vi "Create_Trajectory_Using_TrajectoryLibraryXXX.vi"() -> ()   [LabVIEW 2019]
doc: "This utility creates trajectories based on the robot configuration, constraints and defined waypoints."
uses:
  <vilib>/Rock Robotics/WPI/ThirdParty/JAS_Junk/TrajLib/TypeDef/DISPLAY_WEIGHTED_WAYPOINT.ctl
  <vilib>/Rock Robotics/WPI/ThirdParty/JAS_Junk/TrajLib/TypeDef/TRAJ_STATE.ctl
  <vilib>/Rock Robotics/WPI/ThirdParty/JAS_Junk/TrajLib/TypeDef/POSE2D.ctl
  <vilib>/Rock Robotics/WPI/ThirdParty/JAS_Junk/TrajLib/TypeDef/TRANSLATION2D.ctl
  <vilib>/Rock Robotics/WPI/ThirdParty/JAS_Junk/TrajLib/TypeDef/ROTATION2D.ctl
  <vilib>/Rock Robotics/WPI/ThirdParty/JAS_Junk/TrajLib/TypeDef/SIMPLE_MOTOR_FF.ctl
  CreateTrajectoryENUM/TrajCreateUnitsENUM.ctl
  <vilib>/Rock Robotics/WPI/ThirdParty/JAS_Junk/TrajLib/TypeDef/TRAJECTORY.ctl
  <vilib>/Rock Robotics/WPI/ThirdParty/JAS_Junk/TrajLib/TypeDef/TRAJ_CONFIG.ctl
  <vilib>/vision/Image Controls.llb/IMAQ Image.ctl
  <vilib>/Rock Robotics/WPI/ThirdParty/JAS_Junk/TrajLib/TypeDef/TRAJ_CONSTRAINT_RECT_REGION.ctl
  <vilib>/Rock Robotics/WPI/ThirdParty/JAS_Junk/TrajLib/Enum/TRAJ_CONSTRAINT_TYPES_ENUM.ctl
  <vilib>/Utility/miscctls.llb/LVCursorListTypeDef.ctl
  CreateTrajectoryTypeDef/TrajCreateConfig__V_Internal.ctl
  <vilib>/Rock Robotics/WPI/ThirdParty/JAS_Junk/TrajLib/Conv_Inches_Meters.vi
  <vilib>/Rock Robotics/WPI/ThirdParty/JAS_Junk/TrajLib/Conv_Feet_Meters.vi
  <vilib>/Rock Robotics/WPI/ThirdParty/JAS_Junk/TrajLib/Conv_Meters_Inches.vi
  <vilib>/Rock Robotics/WPI/ThirdParty/JAS_Junk/TrajLib/Conv_Meters_Feet.vi
  <vilib>/Rock Robotics/SystemInterfaces/NetworkCommunication/NetComm_UsageReport_report.vi
  <vilib>/Rock Robotics/WPI/ThirdParty/JAS_Junk/TrajLib/CentripetalAccelConstraint_New.vi
  <vilib>/Rock Robotics/WPI/ThirdParty/JAS_Junk/TrajLib/DiffDriveVoltageConstraint_New.vi
  <vilib>/Rock Robotics/WPI/ThirdParty/JAS_Junk/TrajLib/SwerveDriveKinematicsConstraint_New.vi
  <vilib>/Rock Robotics/WPI/ThirdParty/JAS_Junk/TrajLib/MecaDriveKinematicsConstraint_New.vi
  <vilib>/Rock Robotics/WPI/ThirdParty/JAS_Junk/TrajLib/VI/TrajConstraint_GetType.vi
  <vilib>/Utility/xml.llb/Read From XML File(string).vi
  <vilib>/Utility/Data Type/Get Type Information.vi
  <vilib>/Utility/xml.llb/Write to XML File(string).vi
  <vilib>/Rock Robotics/WPI/ThirdParty/JAS_Junk/TrajLib/Globals/Util_LibraryGlobals.vi
  <vilib>/Rock Robotics/WPI/ThirdParty/JAS_Junk/TrajLib/Trajectory_Library.lvlib
panel:
  out "value":T1={"BottomLeftPoint"={"X"=0.0, "Y"=0.0}, "TopRightPoint"={"X"=0.0, "Y"=0.0}, "Constraint"=variant, "Constraint Type"=enum."DIFF DRIVE KINEMATICS"} {"TopRightPoint"."Y" format="%14.3f"; "TopRightPoint"."X" format="%14.3f"; "BottomLeftPoint"."Y" format="%14.3f"; "BottomLeftPoint"."X" format="%14.3f"}
  out "error out 2":errorcluster
  out "LabVIEW Data":variant
  out "error out":errorcluster
  out "xml string":string
  in  "Terminate":bool
  out "FIeld Image":T4
  out "FIeldSelectorHasItems":bool
  out "IsCubic":bool
  out "outTRAJECTORY_CONFIG":T5 {"End Velocity" format="%20.4f"; "StartVelocity" format="%20.4f"; "Max Acceleration" format="%20.4f"; "MaxVelocity" format="%20.4f"}
  out "WayPoints_M":T6[](array[typedef]) {"WEIGHT" format="%13.3f"; "ANGLE" format="%13.3f"; "Y" format="%13.3f"; "X" format="%13.3f"}
  out "TRAJECTORY":T7 {"States"."POSE"."ROTATION"."SIN" format="%13.4f"; "States"."POSE"."ROTATION"."COS" format="%13.4f"; "States"."POSE"."ROTATION"."VALUE" format="%13.4f"; "States"."POSE"."TRANSLATION"."Y" format="%14.3f"; "States"."POSE"."TRANSLATION"."X" format="%14.3f"; "TotalTImeSecs" format="%20.3f"}
  in  "End Program":bool
  in  "Tab Control":T11(tab)
  out "Config File Read\nWithout Error":bool
  out "Config File  Read Error":errorcluster
  out "Read Config File Comment":string
  in  "Read Config File Name":path
  in  "ReadConfigFile":bool
  in  "Field Selector":string(combo)
  in  "Units Selector":T12
  in  "MaxVelocity":dbl=50.0 format="%17.1f"
  in  "MaxAcceleration":dbl=40.0 format="%17.1f"
  out "MaxVelocity M/S":dbl=2.0 format="%17.4f"
  out "MaxAcceleration M/S^2":dbl=1.3 format="%17.4f"
  in  "Right Rear":T2={"X"=-0.5, "Y"=0.5} {"Y" format="%14.3f"; "X" format="%14.3f"}
  in  "Left Rear":T2={"X"=-0.5, "Y"=-0.5} {"Y" format="%14.3f"; "X" format="%14.3f"}
  in  "Right Front":T2={"X"=0.5, "Y"=0.5} {"Y" format="%14.3f"; "X" format="%14.3f"}
  in  "Left Front":T2={"X"=0.5, "Y"=-0.5} {"Y" format="%14.3f"; "X" format="%14.3f"}
  in  "Use Centripetal\nAcceleration\nConstaint":bool=TRUE
  out "Max Cent Accel M/S^2":dbl=1.0 format="%20.4f"
  in  "Max Cent Accel":dbl=20.0 format="%20.1f"
  in  "Use Diff Drive\nKinematic\nConstraint":bool=TRUE
  out "Track Width M":dbl=0.66 format="%20.4f"
  in  "Track Width":dbl=20.866 format="%20.1f"
  in  "Max Voltage":dbl=12.0 format="%20.4f"
  in  "SIMPLE_MOTOR_FF":T13={"Ks"=0.9, "Kv"=0.22199, "Ka"=0.04876, "KnInv"=1.0} {"KnInv" format="%13.4f"; "Ka" format="%13.4f"; "Kv" format="%13.4f"; "Ks" format="%13.4f"}
  in  "Use Diff Drive\nVoltage\nConstraint":bool
  in  "Wheels":T2[](array[typedef])=[{"X"=0.5, "Y"=-0.5}, {"X"=0.5, "Y"=0.5}, {"X"=-0.5, "Y"=0.5}, {"X"=-0.5, "Y"=-0.5}] {"Y" format="%14.3f"; "X" format="%14.3f"}
  in  "Use Swerve Drive\nKinematics\nConstraint":bool
  in  "Use Mecanum \nDrive Kinematics\nConstraint":bool
  out "Left Front M":T2 {"Y" format="%14.3f"; "X" format="%14.3f"}
  out "Right Front M":T2 {"Y" format="%14.3f"; "X" format="%14.3f"}
  out "Left Rear M":T2 {"Y" format="%14.3f"; "X" format="%14.3f"}
  out "Right Rear M":T2 {"Y" format="%14.3f"; "X" format="%14.3f"}
  out "SIMPLE_MOTOR_FF M":T13={"Ks"=0.0, "Kv"=0.0, "Ka"=0.0, "KnInv"=1.0} {"KnInv" format="%13.4f"; "Ka" format="%13.4f"; "Kv" format="%13.4f"; "Ks" format="%13.4f"}
  out "Wheels M":T2[](array[typedef]) {"Y" format="%14.3f"; "X" format="%14.3f"}
  in  "Use Rectangular Region\nDiff Drive Kinematics\nConstraint":bool
  in  "Rect Reg Top Right":T2 {"Y" format="%14.3f"; "X" format="%14.3f"}
  in  "REct Reg Bot Left":T2 {"Y" format="%14.3f"; "X" format="%14.3f"}
  in  "Max Speed (Units/Sec)":dbl=40.0 format="%20.4f"
  in  "Max Accel (Units/Sec^2)":dbl=100.0 format="%20.4f"
  out "Rect Reg Top Right M":T2 {"Y" format="%14.3f"; "X" format="%14.3f"}
  out "Rect Reg Bot Left M":T2 {"Y" format="%14.3f"; "X" format="%14.3f"}
  out "Max Sped M/Sec":dbl
  out "Max Accel M/Sec^2":dbl
  in  "Remove Current\nWaypoint":bool
  in  "Add New\nWaypoint":bool
  in  "WayPoints":T6[](array[typedef])=[{"X"=15.0, "Y"=105.0, "ANGLE"=-45.0, "WEIGHT"=12.0}, {"X"=105.0, "Y"=65.0, "ANGLE"=0.0, "WEIGHT"=12.0}, {"X"=210.0, "Y"=106.0, "ANGLE"=45.0, "WEIGHT"=12.0}, {"X"=350.0, "Y"=105.0, "ANGLE"=-45.0, "WEIGHT"=12.0}] {"WEIGHT" format="%13.3f"; "ANGLE" format="%13.3f"; "Y" format="%13.3f"; "X" format="%13.3f"}
  in  "Spline Type":enum32{"Radio Selection 1", "Radio Selection 2"}(radio)
  in  "Reverse":bool
  in  "UseWeights":bool
  in  "Calculate\nTrajectory":bool
  out "Trajectory\nCompleted\nError Free":bool
  out "Trajectory calculation error":errorcluster
  out "Position":cluster{dbl[], dbl[]}[](graph)
  out "Field Display":T4(plugin-control)
  out "Index":i32
  out "Trajectory Data":cluster{dbl[], dbl[]}[](graph)
  out "differential \ndrive \nmax speed":dbl format="%15.1f"
  out "Traj States\nSize":i32
  out "Trajectory States":T8[](array[typedef]) {"POSE"."ROTATION"."SIN" format="%13.4f"; "POSE"."ROTATION"."COS" format="%13.4f"; "POSE"."ROTATION"."VALUE" format="%13.4f"; "POSE"."TRANSLATION"."Y" format="%14.3f"; "POSE"."TRANSLATION"."X" format="%14.3f"}
  in  "Trajectory JSON File Name":path
  out "JSON File Saved\nWithout Error":bool
  out "Write CSV File Error":errorcluster
  in  "PathWeaver Length Units":T14(radio)
  in  "WriteJSONFile":bool
  out "CSV File Saved\nWithout Error":bool
  in  "Trajectory Type":enum32{"Radio Selection 1", "Radio Selection 2"}(radio)
  out "Write Trajectory\nFile Error":errorcluster
  in  "Trajectory File Comment":string
  in  "Trajectory CSV File Name":path
  in  "WriteTrajFile":bool
  out "Config File Saved\nWithout Error":bool
  out "Write Config FIle Error":errorcluster
  in  "Write Config File Comment":string
  in  "Write Config File Name":path
  in  "WriteConfigFile":bool
  # "Create Trajectory  (Use LabVIEW trajectory library)"
  # "Instructions:  \n----------------\n\nThis utility will create a trajectory, show the data on the various tabs, and optionally write a \"field absolute\" or \"robot relative\" trajectory to a file. \nTo use this utility:\n\n    1) Read all of these instructions!\n    2) Define the robot's physical data on the \"Robot Data\" tab.  \n    3) Define the robot's movement constraints on the \"Constraints\" page.  \n    4) Define the trajectory on the \"Define/Create Trajectory\" tab.  These are the beginning and ending positions/headings, and internal positions/headings.  \n         Cubic splines only use the first and last \"angle\".  The other internal \"angles\" are calculated.  Quintic splines use all the defined angles.\n    5) Press the \"Calculate Trajectory\".  If a good trajectory was calculated it will be displayed.  If no errors are generated the Trajectory Complete\n         light will be on.  Errors will be displayed in the error indicator.  The path can be recalculated many times before performing any other action.\n\nAfter a Trajectory has been calculated, the \"trajectory can be written to a file.  The absolute path is converted to a robot relative trajectory.  To do this:\n    1) Enter a comment to be included in the file.  Anything can be entered.\n    2) Select the file name.\n    3) Press \"Create Trajectory File\"  If an error occurs it will be displayed in the File Creation Error indicator.\n\nTo:\n  --  Move a WayPoint  -- Left click the waypoint and drag it using the mouse.\n  --  Rotate a WayPoint  -- Left click the waypoint to select, then use the mouse wheel to increase or decrease the heading\n  --  Change WayPoint weight  -- Left click the waypoint to select, then use CTRL key and mouse wheel to increase or decrease the weight.\n\nNotes:\n--------\n- All the robot parameters, path, and field dimensions are in UNITS, and DEGREES.  Select UNITS from the \"Robot Data\" page.  The resulting  \n  trajectory is converted to METERS, and RADIANS to match the rest of this library!\n- The trajectory library is the same as the WPILIB spline and trajectory library for Java and C++.\n- 2019 playing field size - width: 26 ft 11.25 In = 323.25 in , length: 52 ft 5.25 in = 629.25 in  (I didn't verify this for the 2020 version.)\n\nAcknowlegements\n------------------------\n- Nathanael Cornell from FRC team 5205 added the initial code to visually move and rotate waypoints."
  # "Read Trajectory Waypoints and Configuration from File"
  # "ROBOT DATA"
  # "UNITS/SEC"
  # "Meters/SEC"
  # "UNITS/SEC^2"
  # "Meters/SEC^2"
  # "Simulated robot max speed is: 68.266 Inches/Second"
  # "UTILITY CONFIGURATION"
  # "Diff Kinematics Constraint"
  # "Centripetal Accel Constraint"
  # "Diff Voltage Constraint"
  # "UNITS"
  # "UNITS/SEC^2"
  # "VOLTS"
  # "METERS"
  # "METERS/SEC^2"
  # "Distance is:\nUNITS"
  # "Simulated robot wheelbase is 20.87 in"
  # "Ks = Volts\nKv = VoltSec/Meter\nKa = Volt(Sec^2)/Meter"
  # "Swerve Kinematics Constraint"
  # "Mechanum Kinematics Constraint"
  # "Values\nare \nUNITS"
  # "Values\nare \nUNITS"
  # "Rectangular Region Constraint  - Diff Drive Constraint"
  # "Values\nare \nUNITS"
  # "TRAJECTORY DEFINITION"
  # "To delete array elements or the entire array, right click on the array or element, select Data Operations, then select the action to be performed."
  # "UNITS, UNITS, DEGREES, SCALAR"
  # "INCHES/SEC"
  # "Write Trajectory to File   -   CSV, and / or JSON"
  # "Write Trajectory Waypoints and Configuration to File"
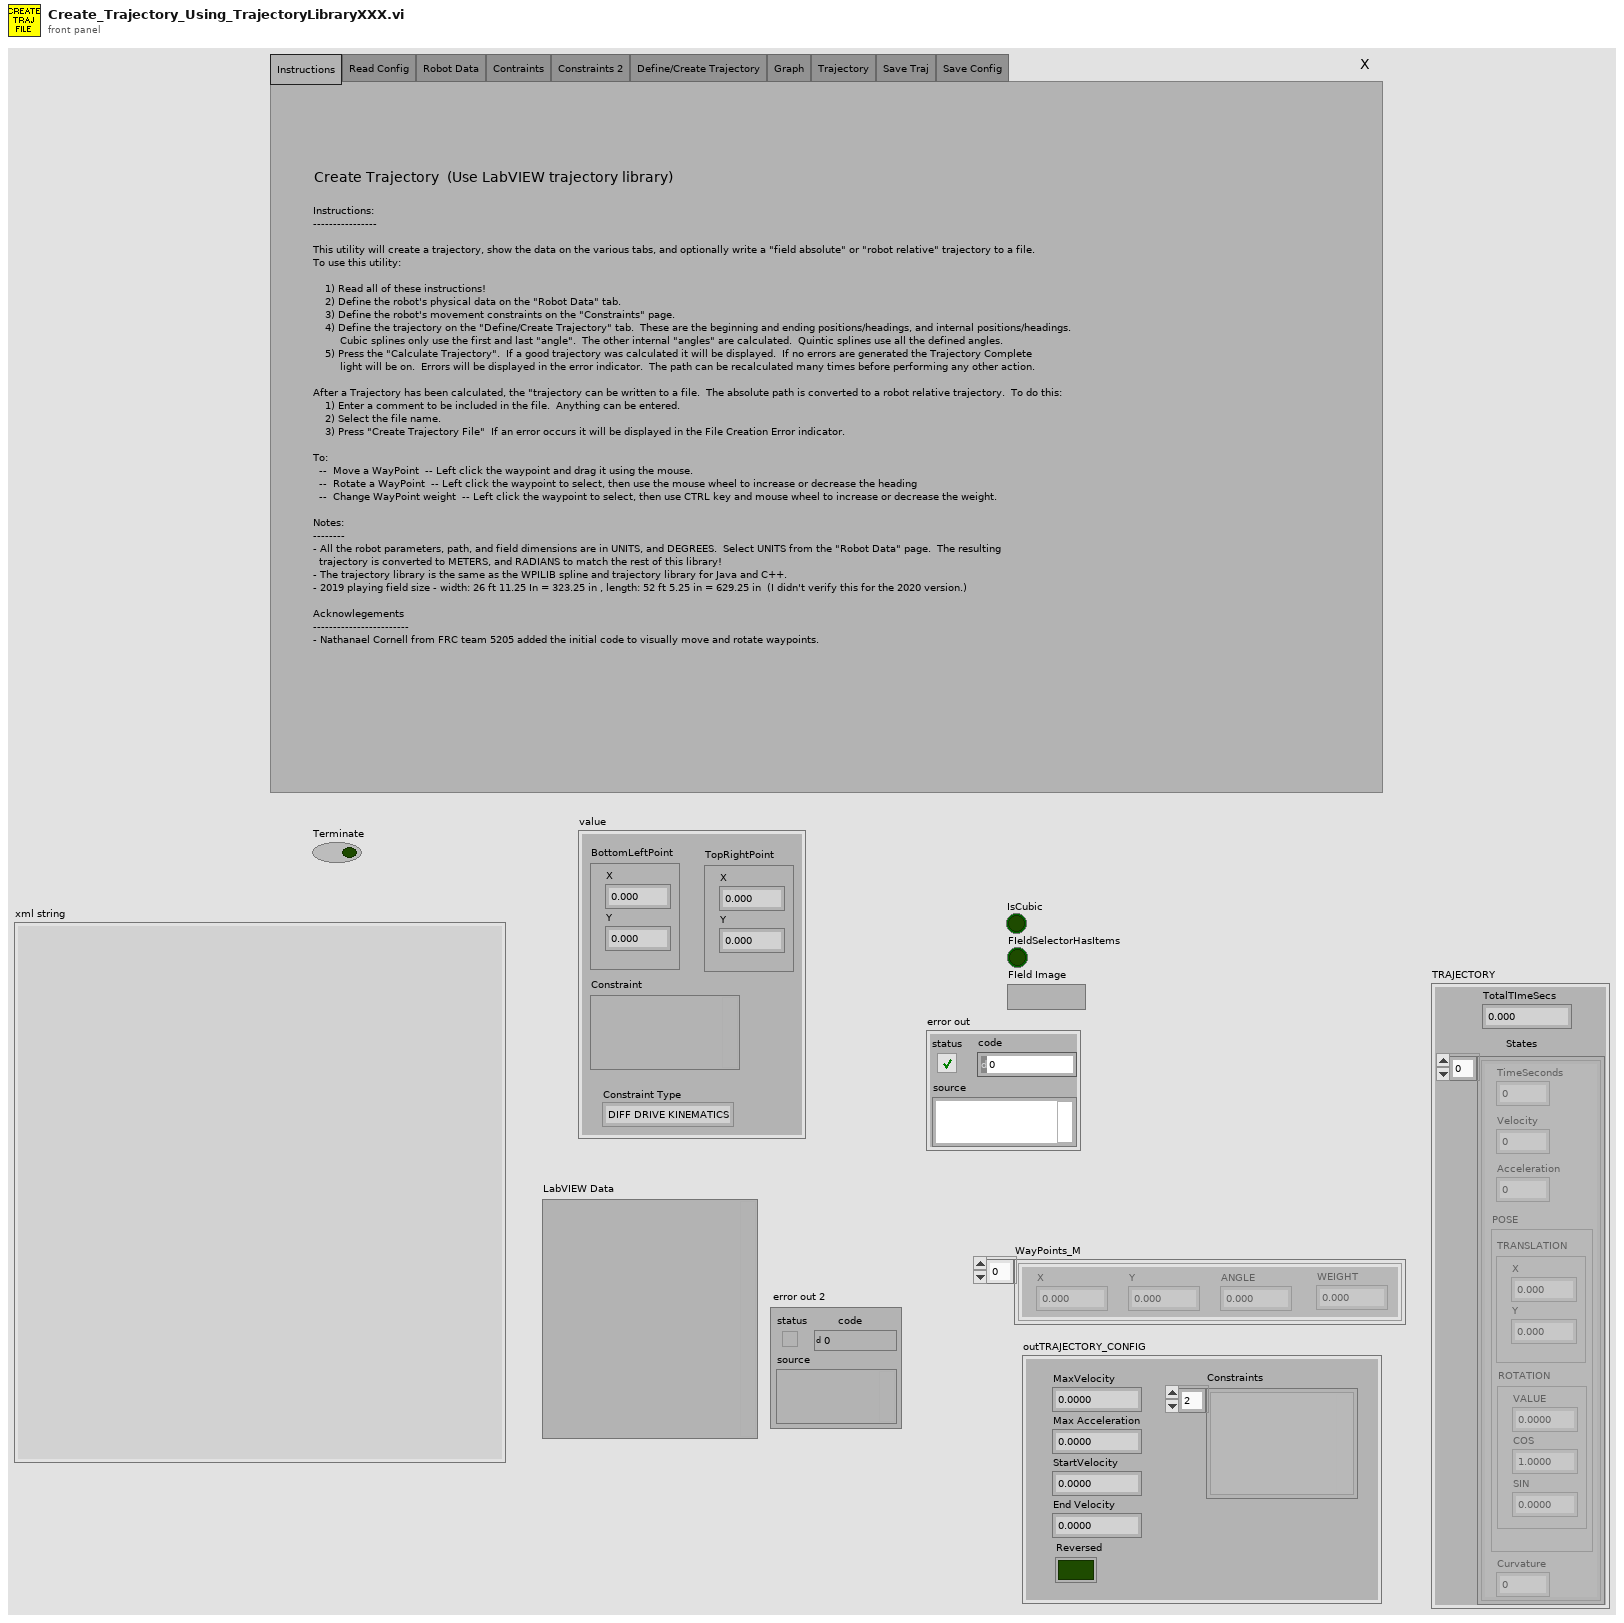
[diagram p1: front panel]
types:
  T1 = typedef "Trajectory_Library.lvlib/TRAJ_CONSTRAINT_RECT_REGION.ctl" = cluster{"BottomLeftPoint":T2, "TopRightPoint":T2, "Constraint":variant, "Constraint Type":T3}
  T2 = typedef "Trajectory_Library.lvlib/TRANSLATION2D.ctl" = cluster{"X":dbl, "Y":dbl}
  T3 = typedef "Trajectory_Library.lvlib/TRAJ_CONSTRAINT_TYPES_ENUM.ctl" = enum16{"UNDEFINED", "DIFF DRIVE KINEMATICS", "DIFF DRIVE VOLTAGE", "CENTRIPITAL ACCEL", "MECA DRIVE KINEMATICS", "SWERVE DRIVE KINEMATICS", "MAXIMUM VELOCITY", "ELLIPTICAL REGION", "RECTANGULAR REGION"}
  T4 = typedef "IMAQ Image.ctl" = refnum<image>
  T5 = typedef "Trajectory_Library.lvlib/TRAJ_CONFIG.ctl" = cluster{"MaxVelocity":dbl, "Max Acceleration":dbl, "StartVelocity":dbl, "End Velocity":dbl, "Reversed":bool, "Constraints":variant[]}
  T6 = typedef "Trajectory_Library.lvlib/DISPLAY_WEIGHTED_WAYPOINT.ctl" = cluster{"X":dbl, "Y":dbl, "ANGLE":dbl, "WEIGHT":dbl}
  T7 = typedef "Trajectory_Library.lvlib/TRAJECTORY.ctl" = cluster{"TotalTImeSecs":dbl, "States":T8[]}
  T8 = typedef "Trajectory_Library.lvlib/TRAJ_STATE.ctl" = cluster{"TimeSeconds":dbl, "Velocity":dbl, "Acceleration":dbl, "POSE":T9, "Curvature":dbl}
  T9 = typedef "Trajectory_Library.lvlib/POSE2D.ctl" = cluster{"TRANSLATION":T2, "ROTATION":T10}
  T10 = typedef "Trajectory_Library.lvlib/ROTATION2D.ctl" = cluster{"VALUE":dbl, "COS":dbl, "SIN":dbl}
  T11 = enum32{"Instructions", "Read Config", "Robot Data", "Contraints", "Constraints 2", "Define/Create Trajectory", "Graph", "Trajectory", "Save Traj", "Save Config"}
  T12 = typedef "TrajCreateUnitsENUM.ctl" = enum16{"Inches", "Feet", "Centimeters", "Meters"}
  T13 = typedef "Trajectory_Library.lvlib/SIMPLE_MOTOR_FF.ctl" = cluster{"Ks":dbl, "Kv":dbl, "Ka":dbl, "KnInv":dbl}
  T14 = enum32{"Radio Selection 1", "Radio Selection 2", "Radio Selection 3", "Radio Selection 4", "Radio Selection 5"}
  T15 = typedef "Image Type" = u32
  T16 = typedef "TrajectoryUtils_Field_Info.ctl" = cluster{"FIeld_File_Name":string, "Top_Left_X":i32, "Top_Left_Y":i32, "Bottom_Right_X":i32, "Bottom_Right_Y":i32, "Field_Size_X":dbl, "Field_Size_Y":dbl, "FIeld_Size_Units":string}
  T17 = typedef "LVCursorListTypeDef.ctl" = cluster{"Name":string, "Color":u32, "Style":u8, "Point Style":u8, "Name Visible":bool, "Allow Drag":bool, "Cursor Mode":u32, "Plot":i32, "Index":i32, "Position":cluster{"X":dbl, "Y":dbl}, "X Scale":u32, "Y Scale":u32, "Watch Plots":i32[], "Watch All Plots":bool, "Plot Area":i32, "Label Offset":cluster{"X":dbl, "Y":dbl}}[]
  T18 = enum8{"Enabled", "Disabled", "Disabled and Grayed Out"}
  T19 = cluster{"Name":string, "Color":u32, "Style":u8, "Point Style":u8, "Name Visible":bool, "Allow Drag":bool, "Cursor Mode":u32, "Plot":i32, "Index":i32, "Position":cluster{"X":dbl, "Y":dbl}, "X Scale":u32, "Y Scale":u32, "Watch Plots":i32[], "Watch All Plots":bool, "Plot Area":i32, "Label Offset":cluster{"X":dbl, "Y":dbl}}
  T20 = typedef "TrajCreateConfig__V_Internal.ctl" = cluster{"Write Config File Name":path, "Write Config File Comment":string, "WayPoints":T6[], "TRAJECTORY_CONFIG":T5, "IsCubic":bool, "Units Selector":T12, "UseWeights":bool, "FieldName":string}
  T21 = typedef "Trajectory_Library.lvlib/TRAJ_CONSTRAINT_DIIF_DRIVE_KINEMATICS.ctl" = cluster{"Max Speed (M/S)":dbl, "DIFF_DRIVE_KINEMATICS":T22, "Max Accel (M/S2)":dbl}
  T22 = typedef "Trajectory_Library.lvlib/DIFF_DRIVE_KINEMATICS.ctl" = cluster{"TrackWidth_Meters":dbl}
  T23 = typedef "Trajectory_Library.lvlib/TRAJ_CONSTRAINT_CENTRIPETAL_ACCEL.ctl" = cluster{"Max Cent Accel":dbl}
  T24 = typedef "Trajectory_Library.lvlib/TRAJ_CONSTRAINT_DIIF_DRIVE_VOLTAGE.ctl" = cluster{"Max Voltage":dbl, "DIFF_DRIVE_KINEMATICS":T22, "SIMPLE_MOTOR_FF":T13}
  T25 = typedef "Trajectory_Library.lvlib/TRAJ_CONSTRAINT_MECA_DRIVE_KINEMATICS.ctl" = cluster{"Max Speed (M/S)":dbl, "MECA_DRIVE_KINEMATICS":T26}
  T26 = typedef "Trajectory_Library.lvlib/MECA_DRIVE_KINEMATICS.ctl" = cluster{"FrontLeft":T2, "FrontRight":T2, "RearLeft":T2, "RearRight":T2, "InverseKinematics":T27, "ForwardKinematics":T27, "PrevCoR":T2}
  T27 = typedef "NI_Matrix.lvlib/RealMatrix.ctl" = dbl[][]
  T28 = typedef "Trajectory_Library.lvlib/TRAJ_CONSTRAINT_SWERVE_DRIVE_KINEMATICS.ctl" = cluster{"Max Speed (M/S)":dbl, "SwerveKinematics":T29}
  T29 = typedef "Trajectory_Library.lvlib/SWERVE_DRIVE_KINEMATICS.ctl" = cluster{"NumModules":i32, "InverseKinematics":T27, "ForwardKinematics":T27, "Modules":T2[], "PrevCoR":T2, "SavedModuleStates":T30[]}
  T30 = typedef "Trajectory_Library.lvlib/SWERVE_DRIVE_MODULE_STATE.ctl" = cluster{"Speed":dbl, "Angle":T10}
  T31 = typedef "TrajCreateConfig_V4.ctl" = cluster{"Write Config File Name":path, "Write Config File Comment":string, "WayPoints":T6[], "TRAJECTORY_CONFIG_V4":T32, "IsCubic":bool, "Units Selector":T12, "UseWeights":bool, "FieldName":string}
  T32 = typedef "TrajCreateTrajConfig_V4.ctl" = cluster{"MaxVelocity":dbl, "Max Acceleration":dbl, "StartVelocity":dbl, "End Velocity":dbl, "Reversed":bool, "DiffDrKineConstntDefined":bool, "CentAcellConstntDefined":bool, "DiffDrVoltConstntDefined":bool, "DIFF_DRIVE_KINE_CONSTRAINT":T21, "CENTRIPETAL_ACCEL_CONSTRAINT":T23, "SwerveDrKineConstntDefined":bool, "SWERVE_DRIVE_KINE_CONSTRAINT":T28, "DIFF_DRIVE_VOLTAGE_CONSTRAINT":T24, "MECANUM_DRIVE_KINE_CONSTRAINT":T25, "MecanumDrKineConstntDefined":bool}
  T33 = cluster{"Shift":bool, "Ctrl":bool, "Alt":bool, "Cmd":bool, "Opt":bool}
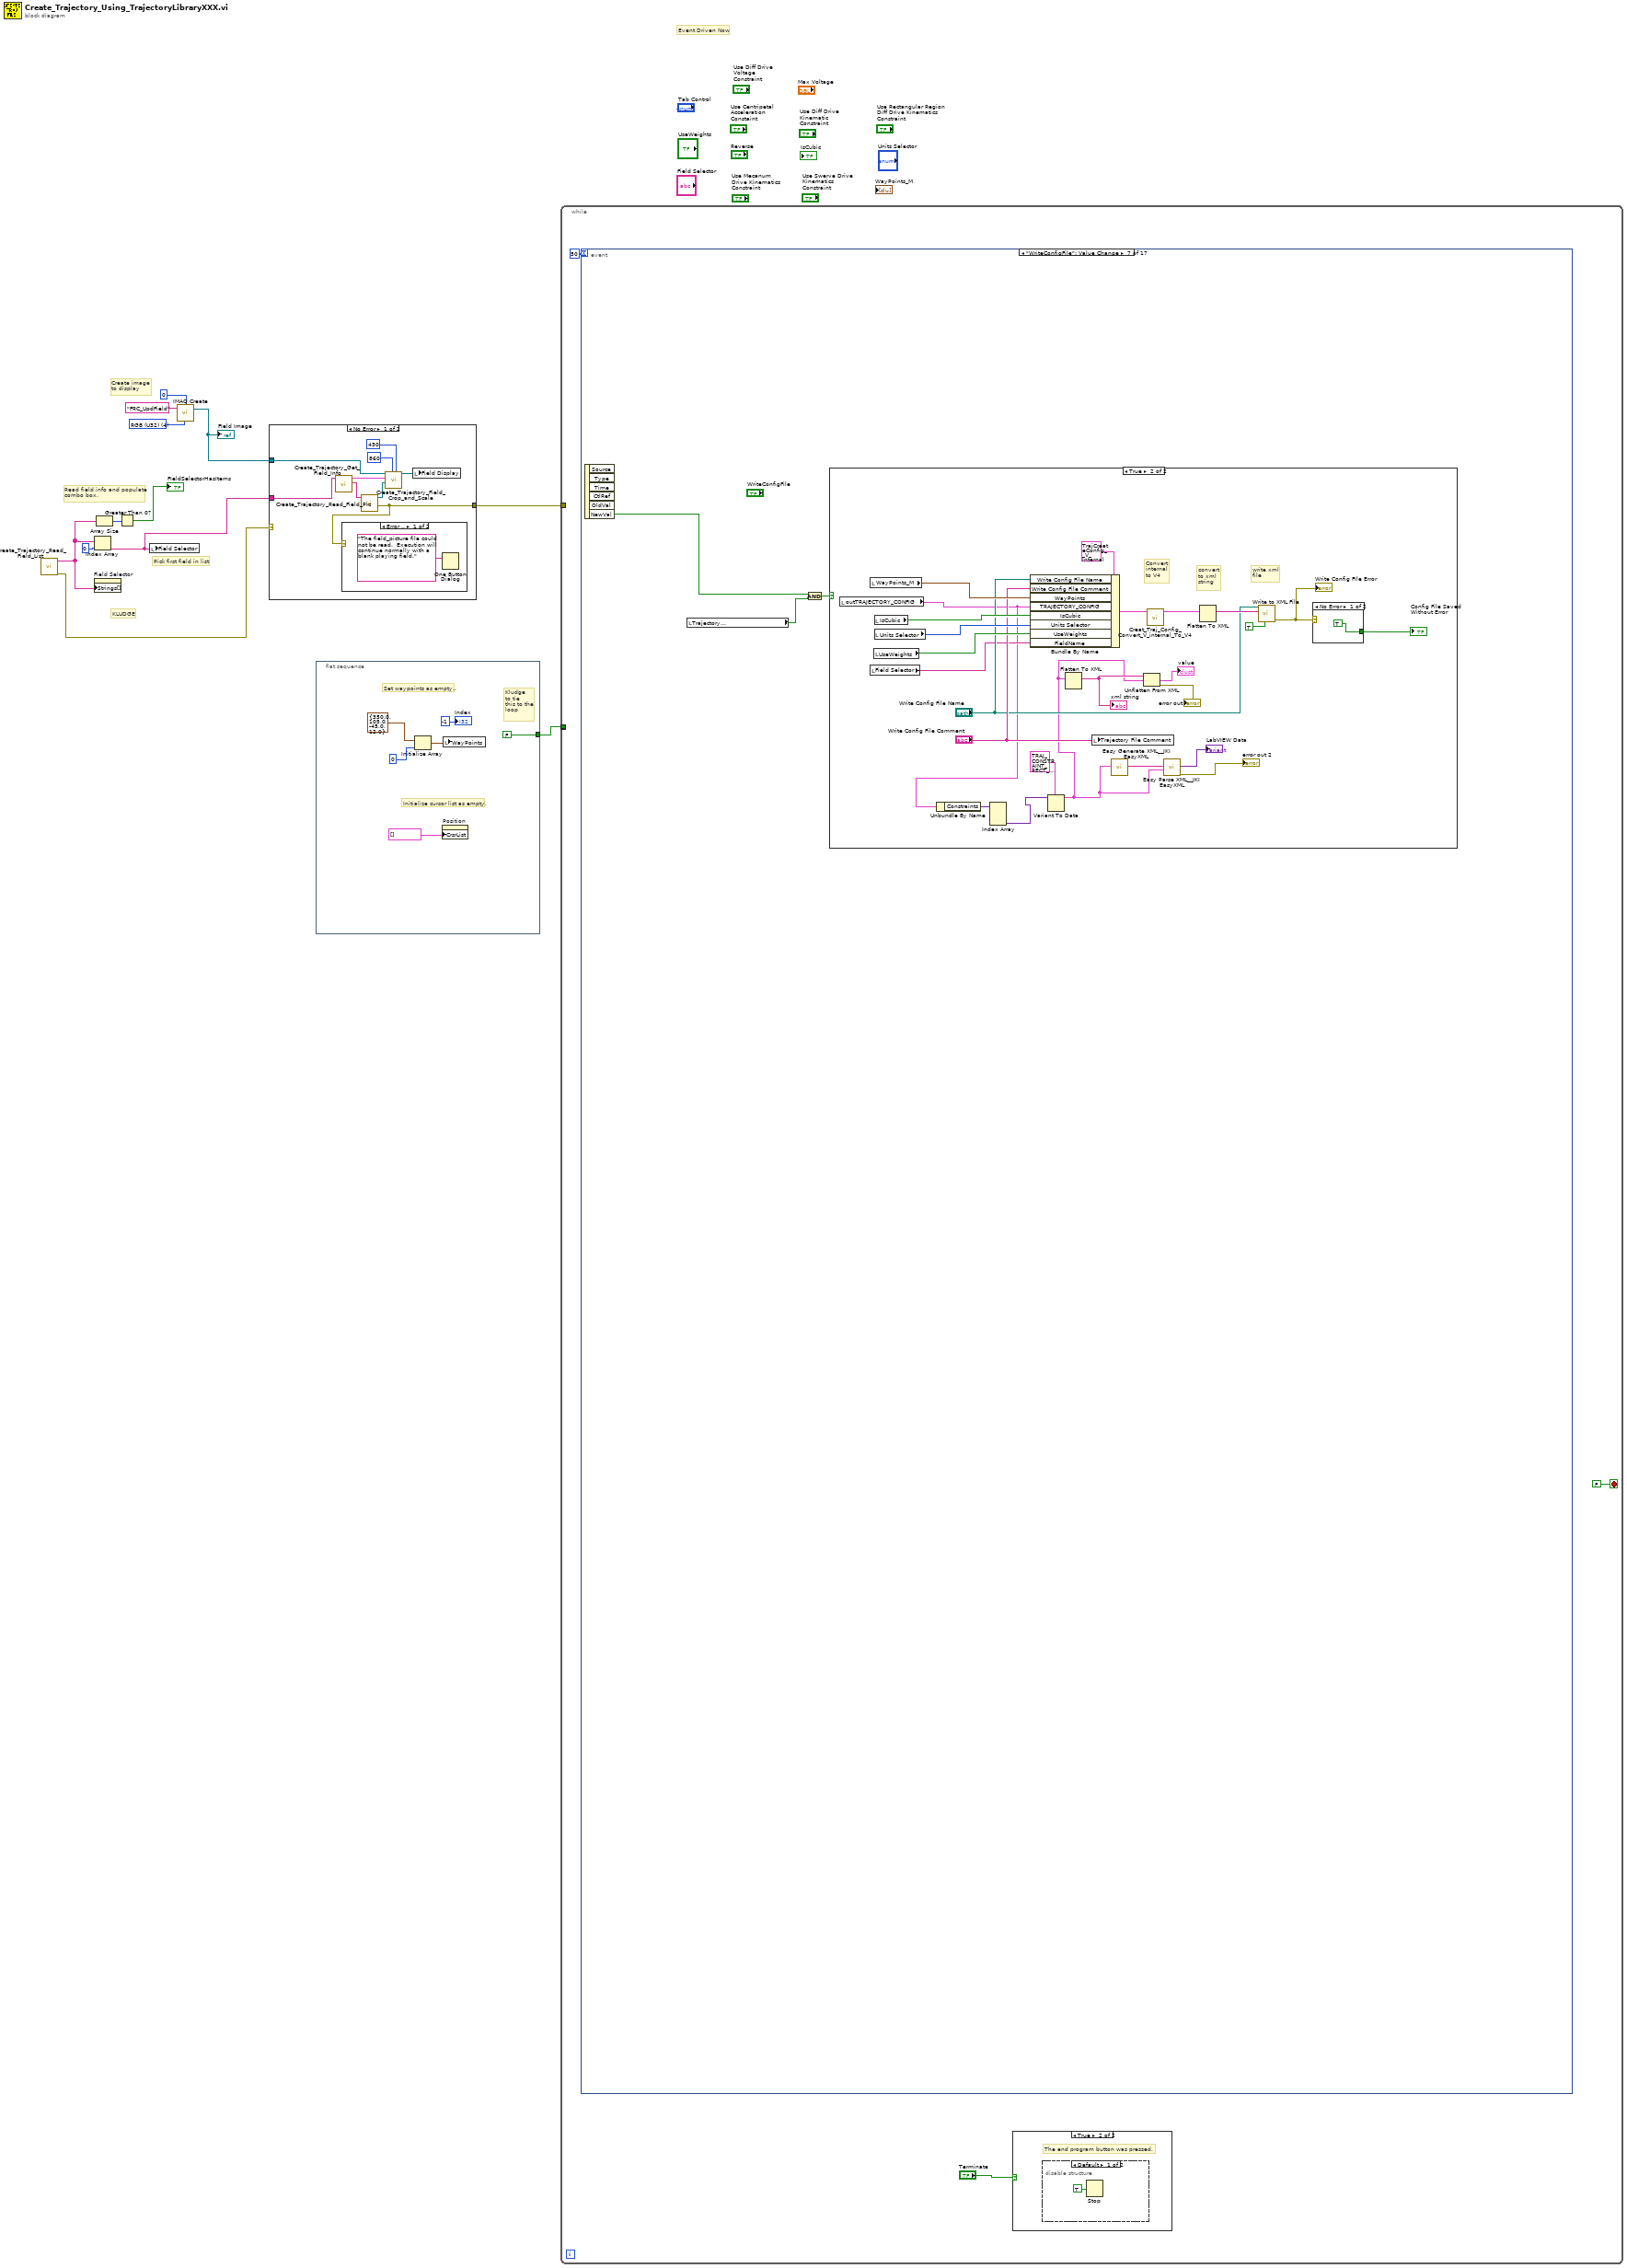
[diagram p0: block diagram]
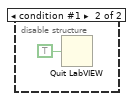
[diagram p3: hidden frame]
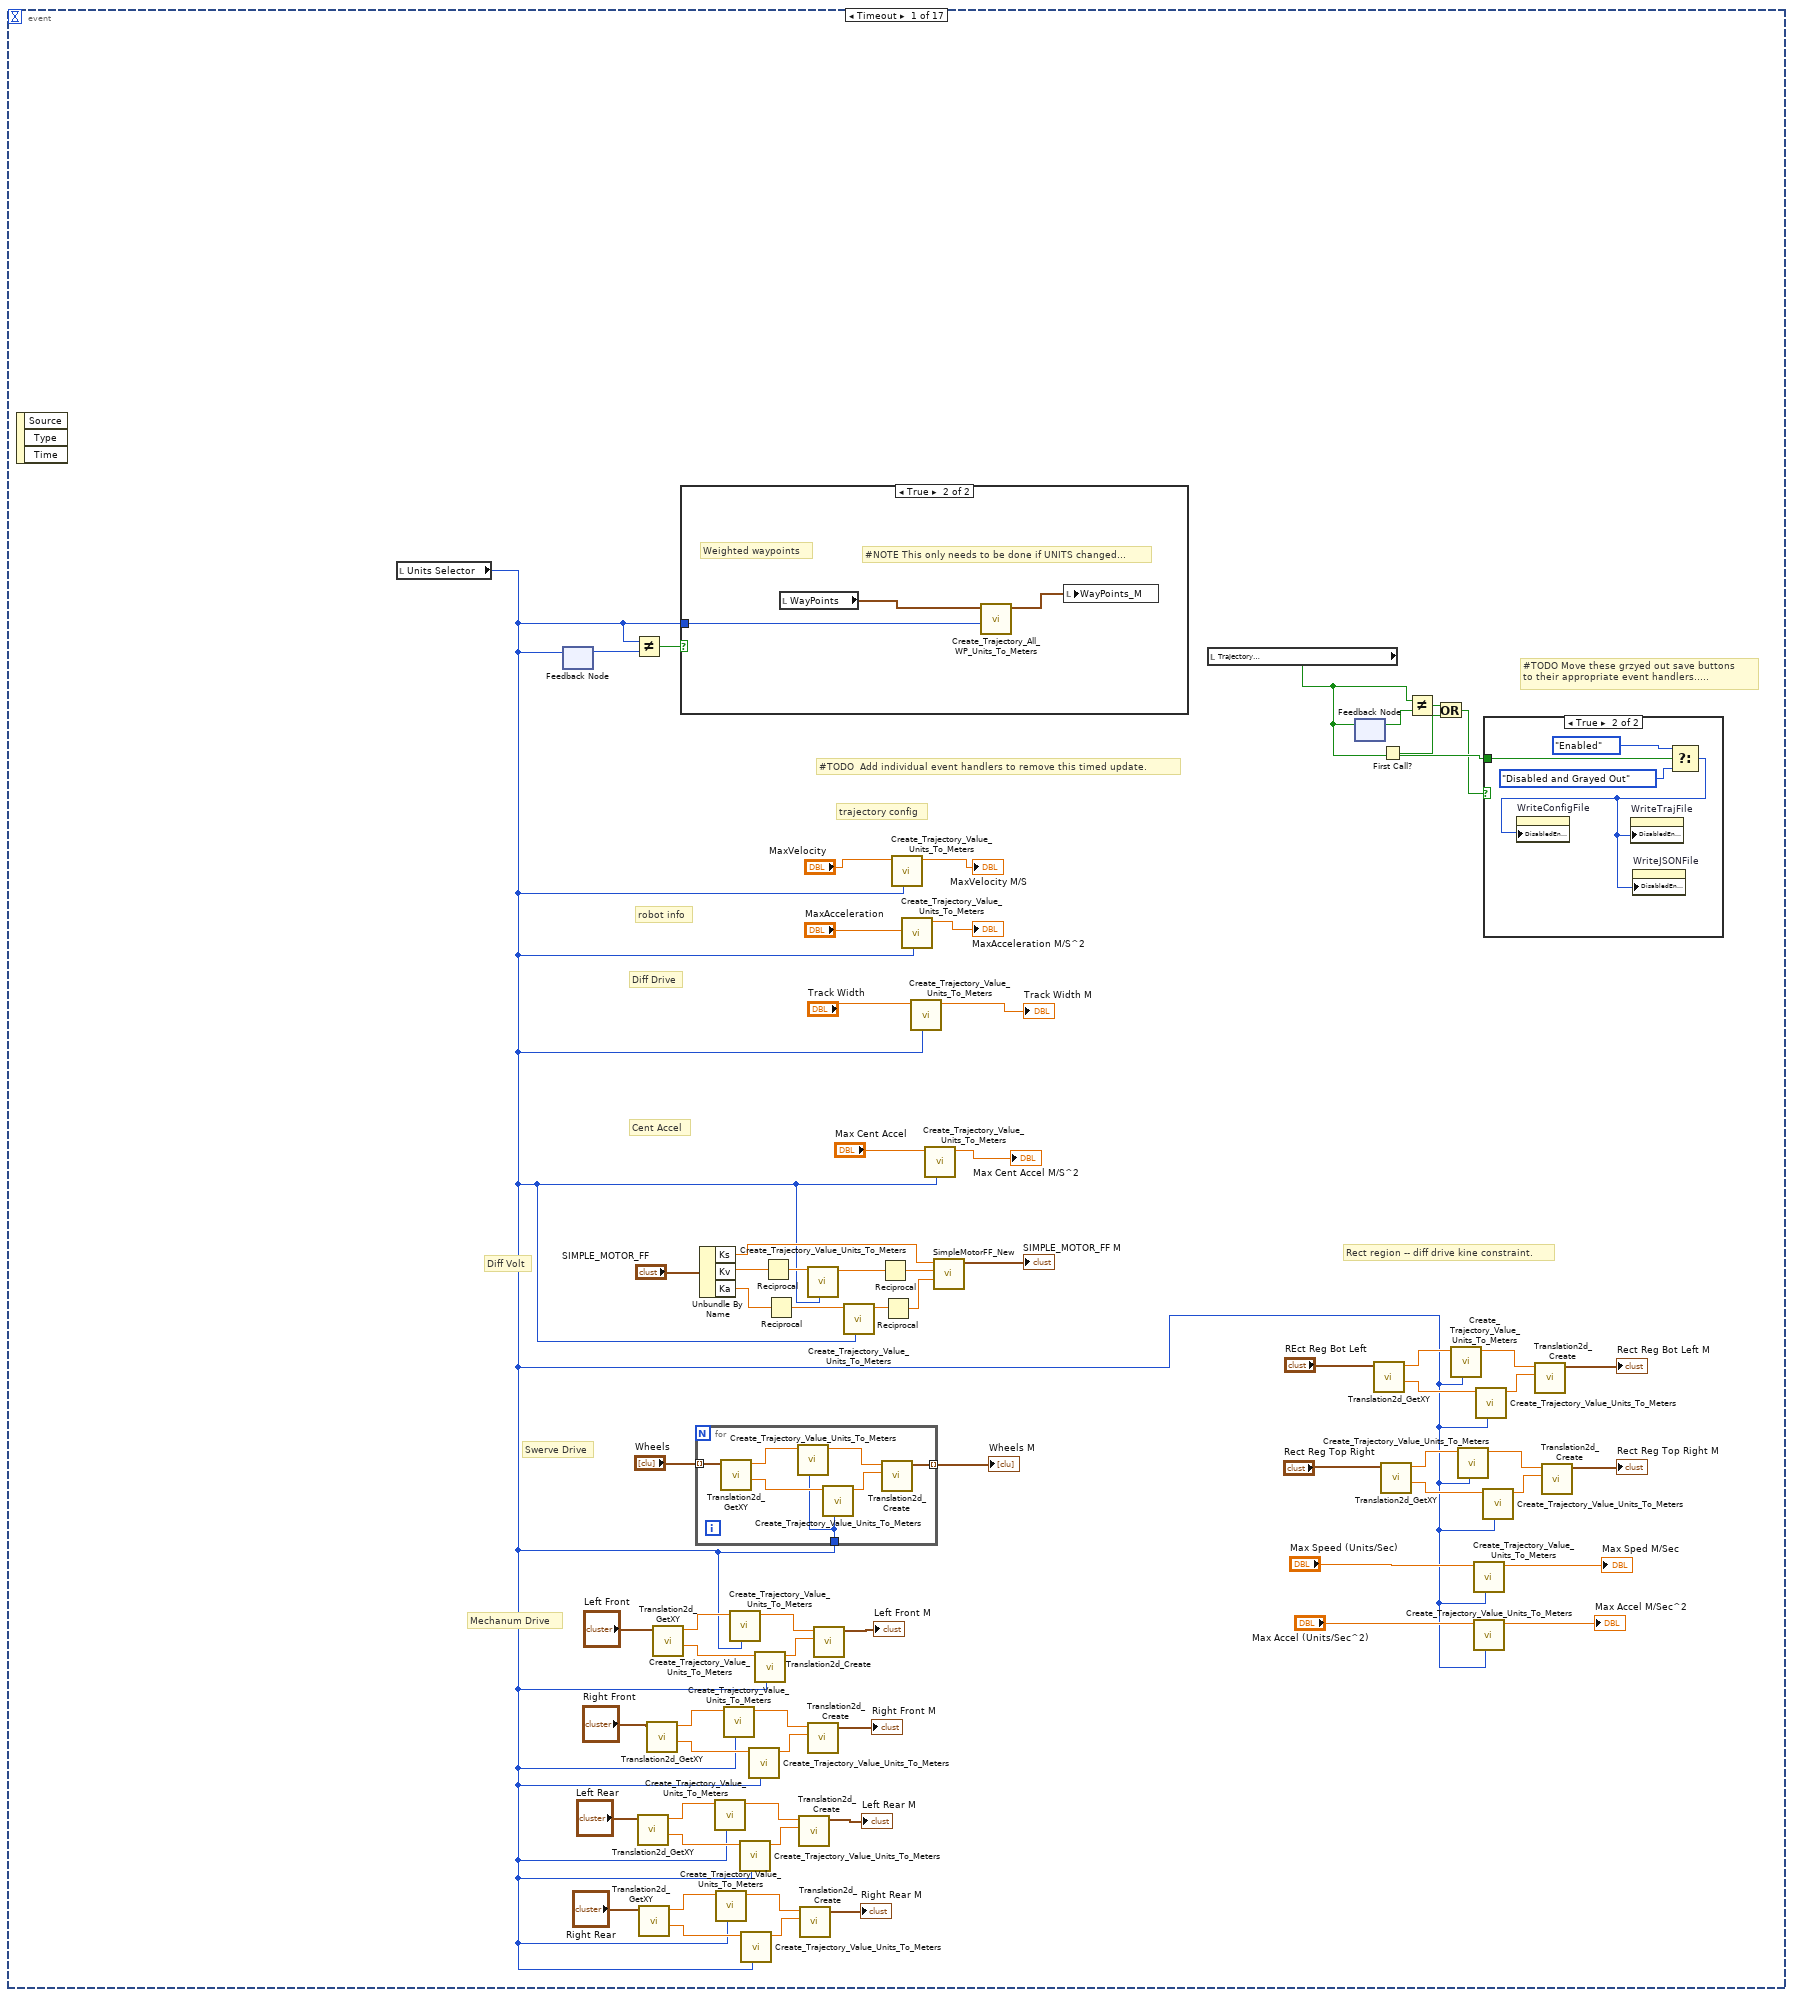
[diagram p4: hidden frame]
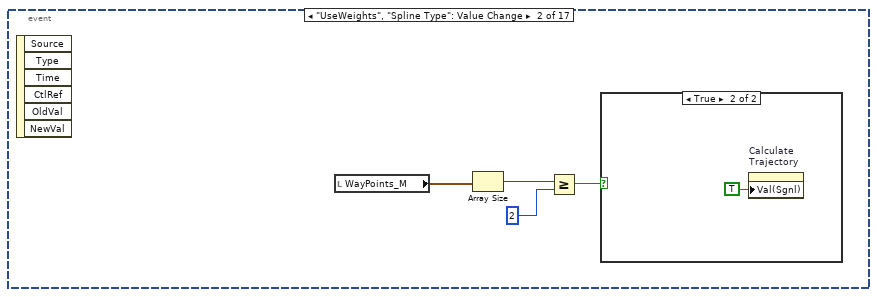
[diagram p7: hidden frame]
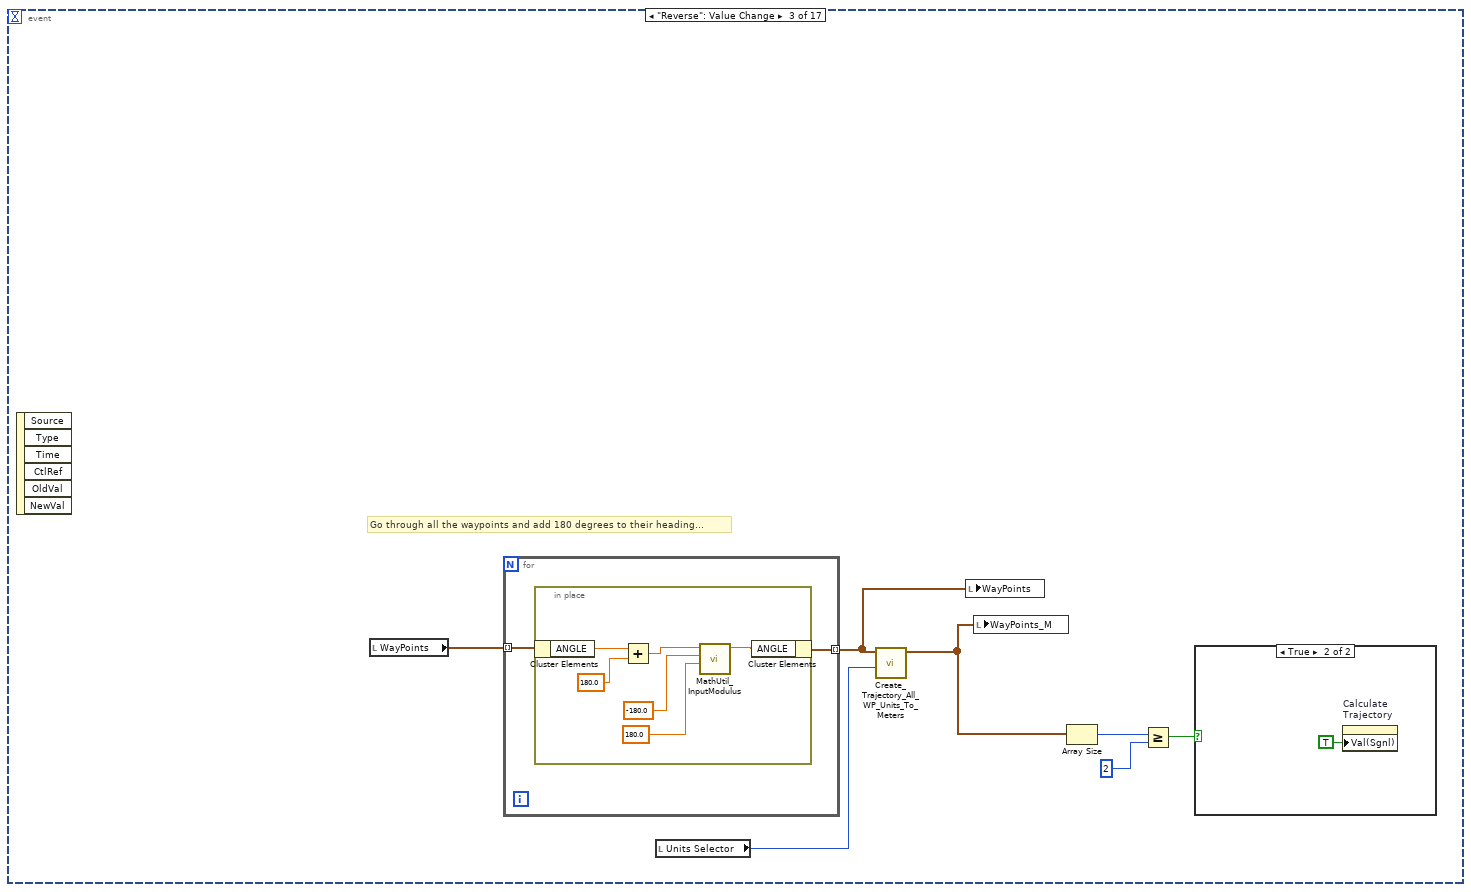
[diagram p9: hidden frame]
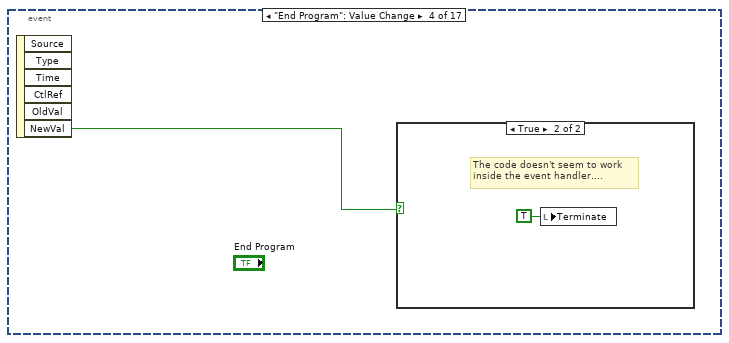
[diagram p11: hidden frame]
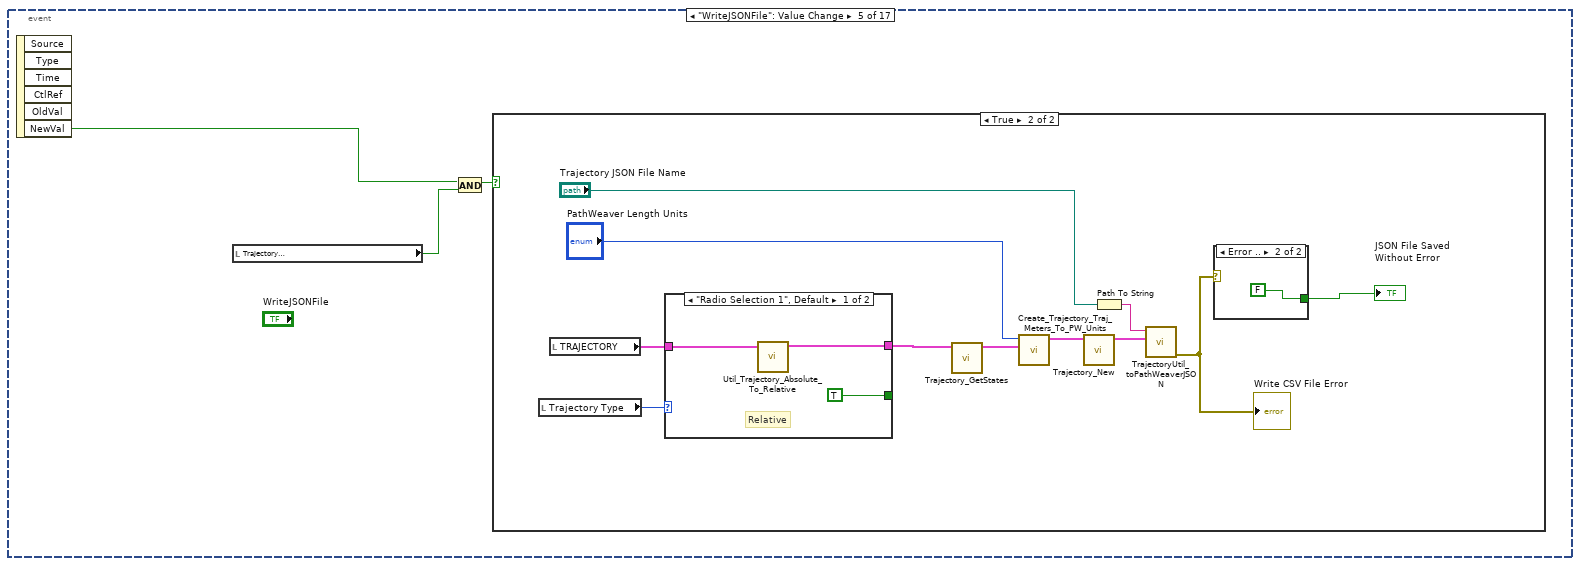
[diagram p13: hidden frame]
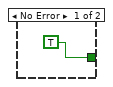
[diagram p15: hidden frame]
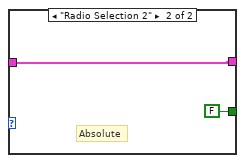
[diagram p16: hidden frame]
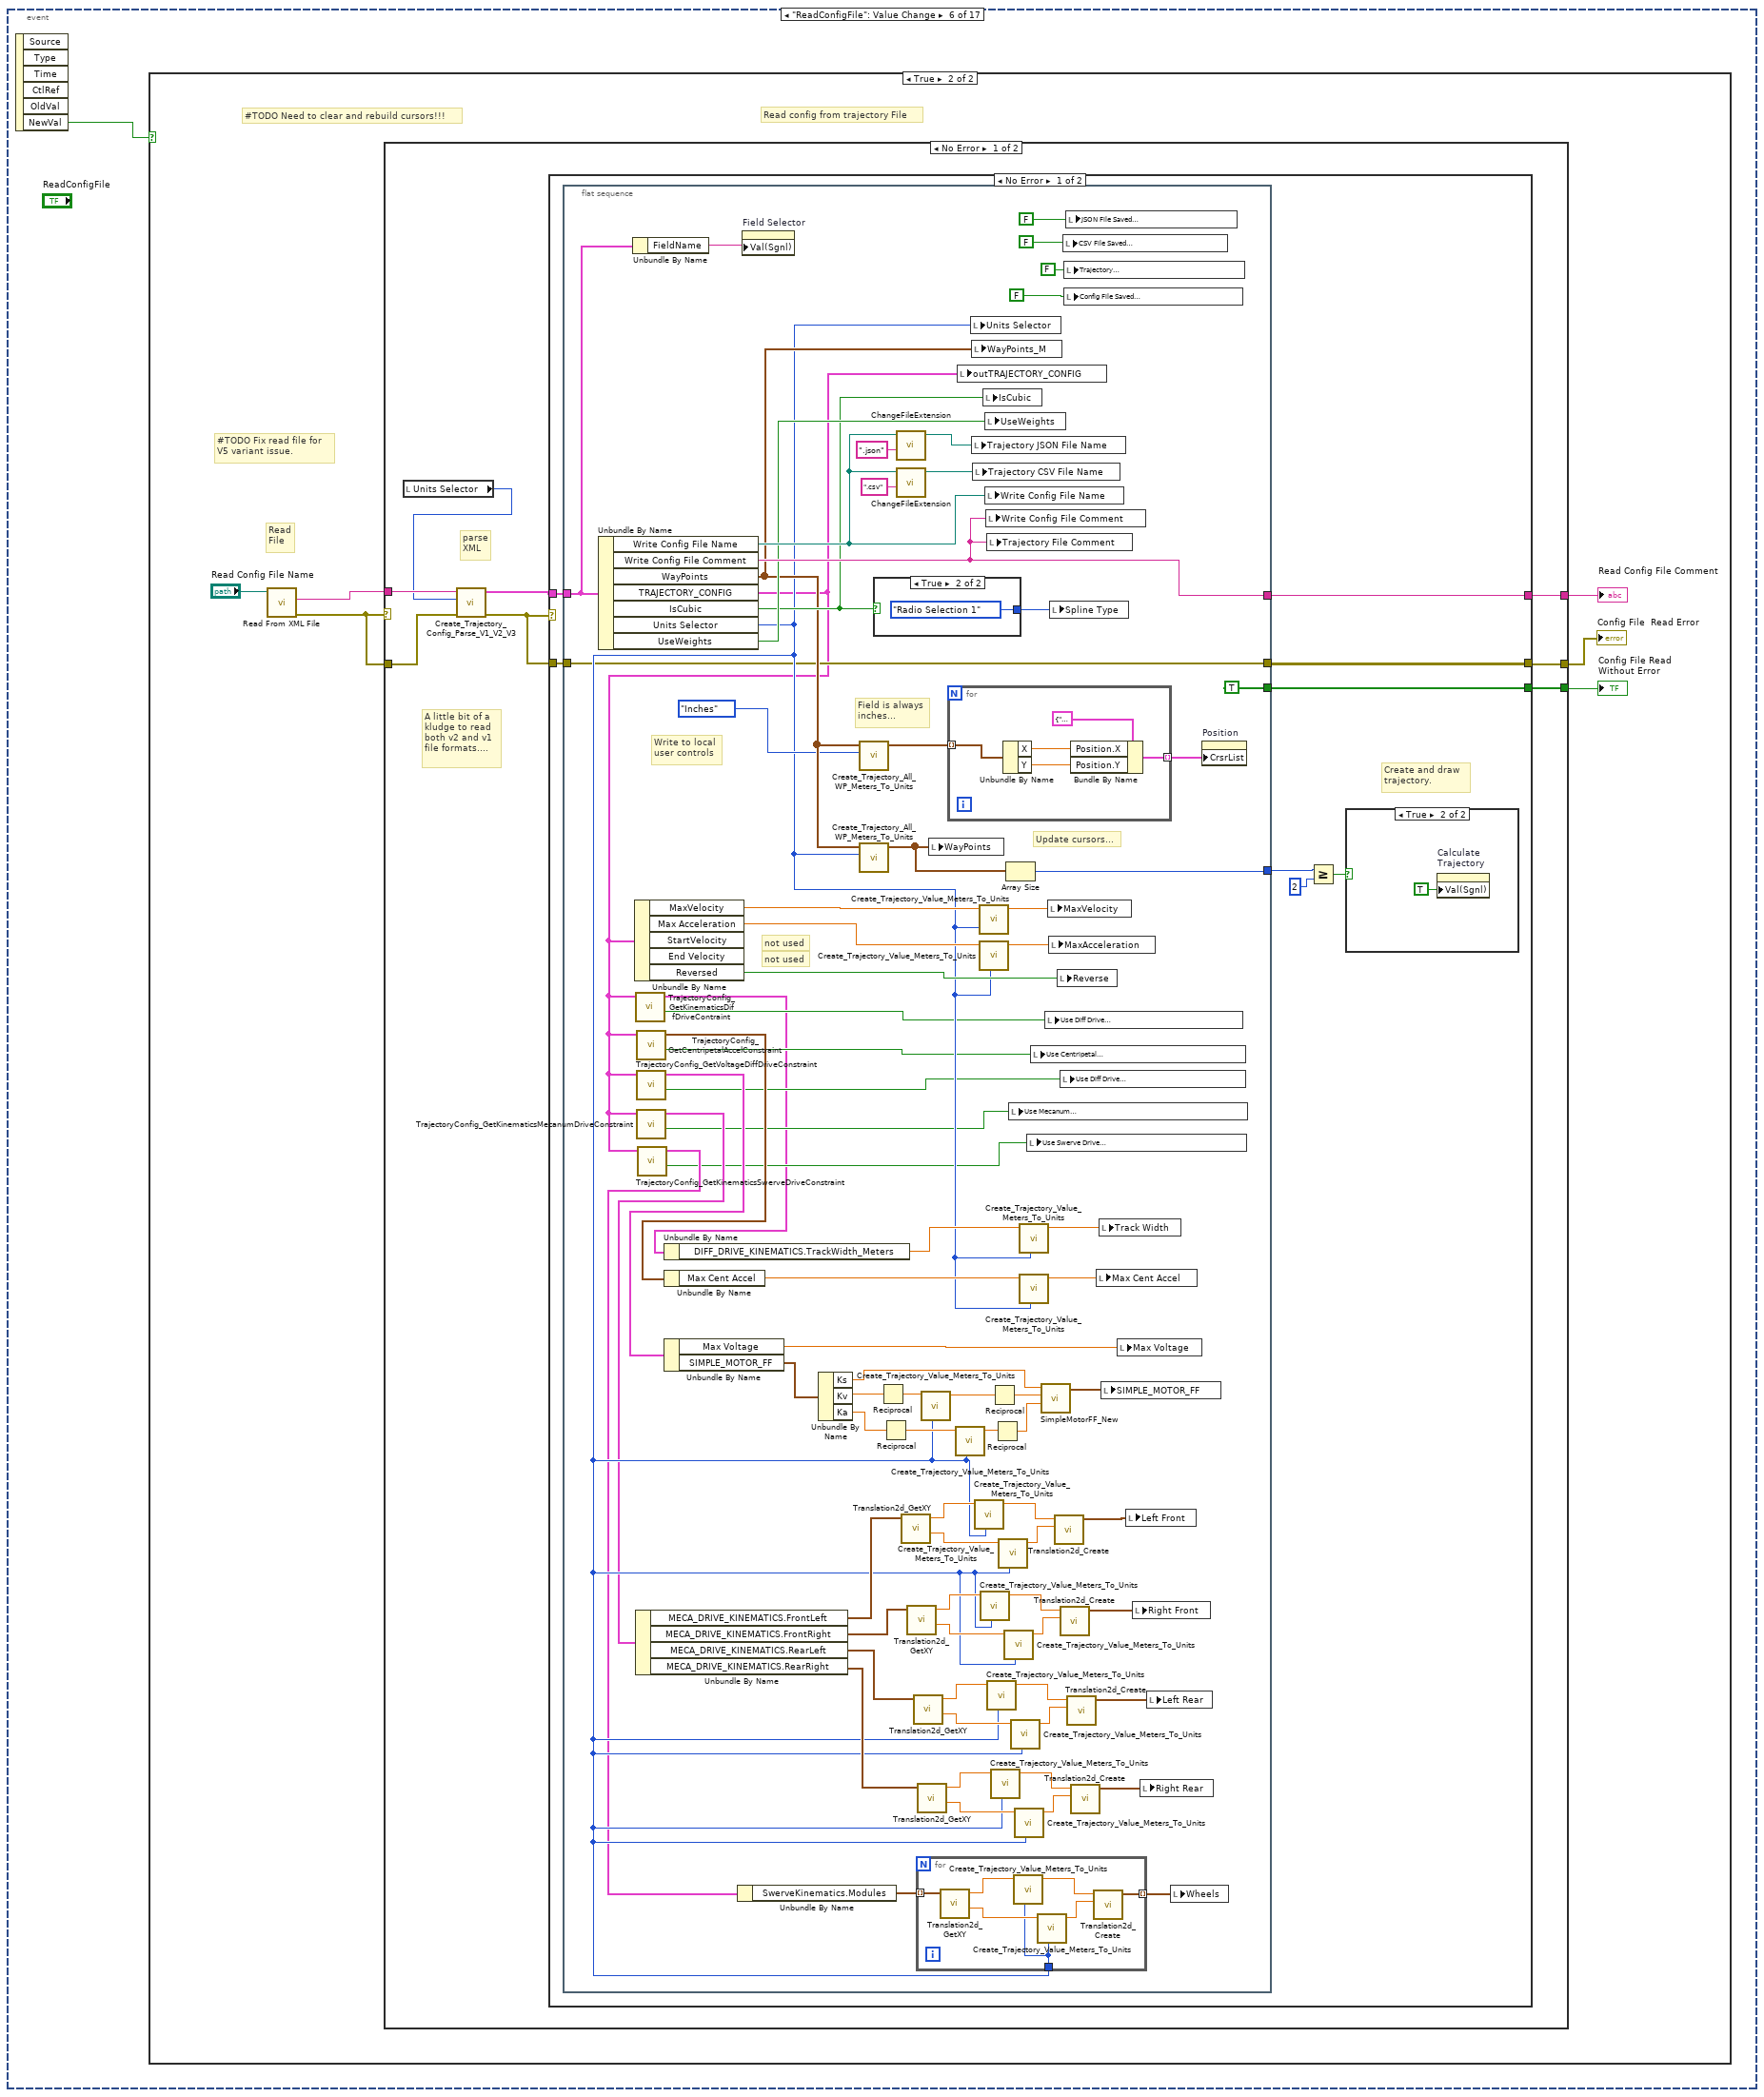
[diagram p17: hidden frame]
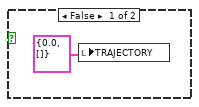
[diagram p19: hidden frame]
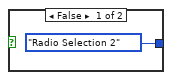
[diagram p20: hidden frame]
diagram:
  w9 = T15 4 items=["Grayscale (U8)", "Grayscale (I16)", "Grayscale (SGL)", "Complex (CSG)", "RGB (U32)", "HSL (U32)", "RGB (U64)", "Grayscale (U16)"] ("Image Type")
  # "Pick first field in list"
  # "Event Driven Now"
  # "Create image \nto display"
  # "KLUDGE"
  # "Read field info and populate\ncombo box."
  n1 = call "Create_Trajectory_Read_Field_List.vi"() -> ("error out"=w6:errorcluster, "section names"=w8:string[])  [unwired: 10 in]
  n2 = property on="Field Selector" class="CmbBox"("Strings[]"=w8) -> ()  [unwired: 2 in, 2 out]
  n3 = Index Array(array=w8, index=0) -> (element=w1:string)
  n4 = Array Size(array=w8) -> (size(s)=w7:i32)
  n5 = Greater Than 0?(x=w7) -> (x > 0?=→"FIeldSelectorHasItems":bool)
  n6 = local write "Field Selector"(w1) -> ()
  n7 = call "IMAQ Create"("Border Size"=0, "Image Name"="FRC_UpdField", "Image Type"=w9) -> ("New Image"=w4:T4)  [unwired: 2 in, 1 out]
  "FIeld Image" <- w4
  n8 = case shown="No Error" w6 {
    selector: w6 -> [_ w23]
    tunnel: w4 -> [w16 _]
    tunnel: [w14 w23] -> w3
    tunnel: w1 -> [w13 _]
    frame No Error {
      n9 = call "Create_Trajectory_Get_Field_Info.vi"("Field Selector"=w13) -> ("File"=w21:string, "input cluster"=w20:T16)  [unwired: 9 in]
      n10 = call "Create_Trajectory_Read_Field_Pic.vi"("file name"=w21) -> ("Image Error"=w14:errorcluster, "Image Data"=w19:T4)  [unwired: 7 in, 2 out]
      n11 = case shown="Error .." w14 {
        frame Error {
          n12 = One Button Dialog(message="The field_picture file could not be read.  Execution will continue normally with a blank playing field.") -> ()  [unwired: 1 in, 1 out]
        }
        frame No Error {
        }
      }
      n13 = call "Create_Trajectory_Field_Crop_and_Scale.vi"("Disp Y Size Pixel"=430, "Disp X Size Pixel"=860, "Field Image"=w19, "field Info"=w20, "Display Image"=w16) -> ("Disp Image Out"=w15:T4)  [unwired: 5 in, 1 out]
      n14 = local write "Field Display"(w15) -> ()
    }
    frame Error {
    }
  }
  n15 = flat-sequence {
    tunnel: [FALSE] -> w2
    frame #0 {
      # "Kludge\nto tie\nthis to the\nloop"
      # "Initialize cursor list as empty."
      # "Set waypoints as empty.."
      n16 = Initialize Array(T6 {"X"=350.0, "Y"=105.0, "ANGLE"=-45.0, "WEIGHT"=12.0} ("path"), 0 ("dimension size")) -> (w27:T6[])
      n17 = property on="Position" class="XYGraph (strict)"("CrsrList"=T17 [] ("Cursor List")) -> ()  [unwired: 2 in, 2 out]
      n18 = local write "WayPoints"(w27) -> ()
      "Index" <- -1 ("Index")
    }
  }
  n19 = while {
    tunnel: w3 -> [_]
    tunnel: [w31] -> _
    tunnel: w2 -> [w31]
    stop <- FALSE stop-if-true
    n20 = event shown="[6] \"WriteConfigFile\": Value Change" {
      selector: _ -> [_ _ _ _ _ _ _ _ _ _ _ _ _ _ _ _ _]
      dyn-events: _ -> [_ _ _ _ _ _ _ _ _ _ _ _ _ _ _ _ _]
      timeout: 50 -> [_ _ _ _ _ _ _ _ _ _ _ _ _ _ _ _ _]
      event Timeout {
        # "Rect region -- diff drive kine constraint."
        # "#TODO  Add individual event handlers to remove this timed update."
        # "#TODO Move these grzyed out save buttons\nto their appropriate event handlers....."
        # "robot info"
        # "Diff Drive"
        # "Cent Accel"
        # "Diff Volt"
        # "Swerve Drive"
        # "Mechanum Drive"
        # "trajectory config"
        n21 = event-data() -> ()  [unwired: 1 in, 3 out]
        n22 = local read "Units Selector"() -> (w41:T12)
        n23 = feedback-in #1(w41) -> ()
        n24 = feedback #1() -> (w54:T12)  [unwired: 1 in]
        n25 = Not Equal?(x=w41, y=w54) -> (x != y?=w55:bool)
        n26 = call <vilib>:"Translation2d_GetXY.vi"("In Translation"="Left Rear") -> ("Y"=w81:dbl, "X"=w79:dbl)  [unwired: 9 in]
        n27 = call <vilib>:"Translation2d_GetXY.vi"("In Translation"="Right Rear") -> ("Y"=w86:dbl, "X"=w84:dbl)  [unwired: 9 in]
        n28 = call <vilib>:"Translation2d_GetXY.vi"("In Translation"="Right Front") -> ("Y"=w76:dbl, "X"=w74:dbl)  [unwired: 9 in]
        n29 = call <vilib>:"Translation2d_GetXY.vi"("In Translation"="Left Front") -> ("Y"=w71:dbl, "X"=w68:dbl)  [unwired: 9 in]
        n30 = case shown="True" w55 {
          tunnel: w41 -> [_ w107]
          frame False {
          }
          frame True {
            # "#NOTE This only needs to be done if UNITS changed..."
            # "Weighted waypoints"
            n31 = local read "WayPoints"() -> (w105:T6[])
            n32 = call "Create_Trajectory_All_WP_Units_To_Meters.vi"("Units Selector"=w107, "WayPoints"=w105) -> ("Array"=w106:T6[])  [unwired: 9 in]
            n33 = local write "WayPoints_M"(w106) -> ()
          }
        }
        n34 = for {
          tunnel: "Wheels" -> [w114] mode=indexing
          tunnel: [w113] -> w104 mode=indexing
          tunnel: w41 -> [w112]
          n35 = call <vilib>:"Translation2d_GetXY.vi"("In Translation"=w114) -> ("Y"=w116:dbl, "X"=w118:dbl)  [unwired: 9 in]
          n36 = call "Create_Trajectory_Value_Units_To_Meters.vi"("Units Selector"=w112, "Units"=w118) -> ("Meters"=w117:dbl)  [unwired: 9 in]
          n37 = call "Create_Trajectory_Value_Units_To_Meters.vi"("Units Selector"=w112, "Units"=w116) -> ("Meters"=w115:dbl)  [unwired: 9 in]
          n38 = call <vilib>:"Translation2d_Create.vi"("Y"=w115, "X"=w117) -> ("TRANSLATION"=w113:T2)  [unwired: 9 in]
        }
        "Wheels M" <- w104
        n39 = Unbundle By Name("SIMPLE_MOTOR_FF") -> ("Ks"=w94:dbl, "Kv"=w95:dbl, "Ka"=w102:dbl)
        n40 = call "Create_Trajectory_Value_Units_To_Meters.vi"("Units Selector"=w41, "Units"=w79) -> ("Meters"=w80:dbl)  [unwired: 9 in]
        n41 = call "Create_Trajectory_Value_Units_To_Meters.vi"("Units Selector"=w41, "Units"=w84) -> ("Meters"=w85:dbl)  [unwired: 9 in]
        n42 = call "Create_Trajectory_Value_Units_To_Meters.vi"("Units Selector"=w41, "Units"=w74) -> ("Meters"=w75:dbl)  [unwired: 9 in]
        n43 = call "Create_Trajectory_Value_Units_To_Meters.vi"("Units Selector"=w41, "Units"=w68) -> ("Meters"=w69:dbl)  [unwired: 9 in]
        n44 = call "Create_Trajectory_Value_Units_To_Meters.vi"("Units Selector"=w41, "Units"=w81) -> ("Meters"=w82:dbl)  [unwired: 9 in]
        n45 = call "Create_Trajectory_Value_Units_To_Meters.vi"("Units Selector"=w41, "Units"=w86) -> ("Meters"=w87:dbl)  [unwired: 9 in]
        n46 = call "Create_Trajectory_Value_Units_To_Meters.vi"("Units Selector"=w41, "Units"=w76) -> ("Meters"=w77:dbl)  [unwired: 9 in]
        n47 = call "Create_Trajectory_Value_Units_To_Meters.vi"("Units Selector"=w41, "Units"=w71) -> ("Meters"=w72:dbl)  [unwired: 9 in]
        n48 = Reciprocal(x=w95) -> (1/x=w96:dbl)
        n49 = Reciprocal(x=w102) -> (1/x=w99:dbl)
        n50 = call <vilib>:"Translation2d_Create.vi"("Y"=w82, "X"=w80) -> ("TRANSLATION"=→"Left Rear M":T2)  [unwired: 9 in]
        n51 = call <vilib>:"Translation2d_Create.vi"("Y"=w87, "X"=w85) -> ("TRANSLATION"=→"Right Rear M":T2)  [unwired: 9 in]
        n52 = call "Create_Trajectory_Value_Units_To_Meters.vi"("Units Selector"=w41, "Units"=w96) -> ("Meters"=w97:dbl)  [unwired: 9 in]
        n53 = call <vilib>:"Translation2d_Create.vi"("Y"=w77, "X"=w75) -> ("TRANSLATION"=→"Right Front M":T2)  [unwired: 9 in]
        n54 = call <vilib>:"Translation2d_Create.vi"("Y"=w72, "X"=w69) -> ("TRANSLATION"=→"Left Front M":T2)  [unwired: 9 in]
        n55 = call "Create_Trajectory_Value_Units_To_Meters.vi"("Units Selector"=w41, "Units"=w99) -> ("Meters"=w100:dbl)  [unwired: 9 in]
        n56 = Reciprocal(x=w97) -> (1/x=w98:dbl)
        n57 = Reciprocal(x=w100) -> (1/x=w101:dbl)
        n58 = call "Create_Trajectory_Value_Units_To_Meters.vi"("Units Selector"=w41, "Units"="MaxVelocity") -> ("Meters"=→"MaxVelocity M/S":dbl)  [unwired: 9 in]
        n59 = call "Create_Trajectory_Value_Units_To_Meters.vi"("Units Selector"=w41, "Units"="MaxAcceleration") -> ("Meters"=→"MaxAcceleration M/S^2":dbl)  [unwired: 9 in]
        n60 = call "Create_Trajectory_Value_Units_To_Meters.vi"("Units Selector"=w41, "Units"="Track Width") -> ("Meters"=→"Track Width M":dbl)  [unwired: 9 in]
        n61 = call "Create_Trajectory_Value_Units_To_Meters.vi"("Units Selector"=w41, "Units"="Max Cent Accel") -> ("Meters"=→"Max Cent Accel M/S^2":dbl)  [unwired: 9 in]
        n62 = call <vilib>:"SimpleMotorFF_New.vi"("Ka"=w101, "Kv"=w98, "Ks"=w94) -> ("SIMPLE_MOTOR_FF"=→"SIMPLE_MOTOR_FF M":T13)  [unwired: 8 in]
        n63 = local read "Trajectory\nCompleted\nError Free"() -> (w60:bool)
        n64 = feedback #2() -> (w56:bool)  [unwired: 1 in]
        n65 = feedback-in #2(w60) -> ()
        n66 = call <vilib>:"Translation2d_GetXY.vi"("In Translation"="REct Reg Bot Left") -> ("Y"=w51:dbl, "X"=w49:dbl)  [unwired: 9 in]
        n67 = First Call?() -> (First Call?: T/F=w58:bool)
        n68 = call <vilib>:"Translation2d_GetXY.vi"("In Translation"="Rect Reg Top Right") -> ("Y"=w47:dbl, "X"=w45:dbl)  [unwired: 9 in]
        n69 = Not Equal?(x=w60, y=w56) -> (x != y?=w57:bool)
        n70 = Or(x=w57, y=w58) -> (x .or. y?=w59:bool)
        n71 = call "Create_Trajectory_Value_Units_To_Meters.vi"("Units Selector"=w41, "Units"=w49) -> ("Meters"=w50:dbl)  [unwired: 9 in]
        n72 = call "Create_Trajectory_Value_Units_To_Meters.vi"("Units Selector"=w41, "Units"=w45) -> ("Meters"=w46:dbl)  [unwired: 9 in]
        n73 = call "Create_Trajectory_Value_Units_To_Meters.vi"("Units Selector"=w41, "Units"="Max Speed (Units/Sec)") -> ("Meters"=→"Max Sped M/Sec":dbl)  [unwired: 9 in]
        n74 = call "Create_Trajectory_Value_Units_To_Meters.vi"("Units Selector"=w41, "Units"="Max Accel (Units/Sec^2)") -> ("Meters"=→"Max Accel M/Sec^2":dbl)  [unwired: 9 in]
        n75 = call "Create_Trajectory_Value_Units_To_Meters.vi"("Units Selector"=w41, "Units"=w51) -> ("Meters"=w52:dbl)  [unwired: 9 in]
        n76 = call "Create_Trajectory_Value_Units_To_Meters.vi"("Units Selector"=w41, "Units"=w47) -> ("Meters"=w48:dbl)  [unwired: 9 in]
        n77 = case shown="True" w59 {
          tunnel: w60 -> [_ w111]
          frame False {
          }
          frame True {
            n78 = Select(t=T18."Enabled" ("Disabled"), s=w111, f=T18."Disabled and Grayed Out" ("Disabled")) -> (s? t:f=w108:T18)
            n79 = property on="WriteConfigFile" class="Bool"("DisabledEnum"=w108) -> ()  [unwired: 2 in, 2 out]
            n80 = property on="WriteTrajFile" class="Bool"("DisabledEnum"=w108) -> ()  [unwired: 2 in, 2 out]
            n81 = property on="WriteJSONFile" class="Bool"("DisabledEnum"=w108) -> ()  [unwired: 2 in, 2 out]
          }
        }
        n82 = call <vilib>:"Translation2d_Create.vi"("Y"=w52, "X"=w50) -> ("TRANSLATION"=→"Rect Reg Bot Left M":T2)  [unwired: 9 in]
        n83 = call <vilib>:"Translation2d_Create.vi"("Y"=w48, "X"=w46) -> ("TRANSLATION"=→"Rect Reg Top Right M":T2)  [unwired: 9 in]
      }
      event "UseWeights", "Spline Type": Value Change {
        n84 = event-data() -> ()  [unwired: 1 in, 6 out]
        n85 = local read "WayPoints_M"() -> (w122:T6[])
        n86 = Array Size(array=w122) -> (size(s)=w121:i32)
        n87 = Greater Or Equal?(x=w121, y=2) -> (x >= y?=w119:bool)
        n88 = case shown="True" w119 {
          frame False {
          }
          frame True {
            n89 = property on="Calculate\nTrajectory" class="Bool (strict)"("Val(Sgnl)"=TRUE ("Value (Signaling)")) -> ()  [unwired: 2 in, 2 out]
          }
        }
      }
      event "Reverse": Value Change {
        # "Go through all the waypoints and add 180 degrees to their heading..."
        n90 = event-data() -> ()  [unwired: 1 in, 6 out]
        n91 = local read "WayPoints"() -> (w126:T6[])
        n92 = for {
          tunnel: w126 -> [w132] mode=indexing
          tunnel: [w131] -> w125 mode=indexing
          n93 = in-place {
            n94 = in-place-cluster #3(w132) -> ("ANGLE"=w138:dbl)
            n95 = Add(x=w138, y=180.0) -> (x+y=w134:dbl)
            n96 = call <vilib>:"MathUtil_InputModulus.vi"("Maximum_Input"=180.0, "Minimum_Input"=-180.0, "Input"=w134) -> ("modulus"=w133:dbl)  [unwired: 8 in]
            n97 = in-place-cluster #3("ANGLE"=w133) -> (w131:T6)
          }
        }
        n98 = local read "Units Selector"() -> (w124:T12)
        n99 = call "Create_Trajectory_All_WP_Units_To_Meters.vi"("Units Selector"=w124, "WayPoints"=w125) -> ("Array"=w127:T6[])  [unwired: 9 in]
        n100 = local write "WayPoints"(w125) -> ()
        n101 = local write "WayPoints_M"(w127) -> ()
        n102 = Array Size(array=w127) -> (size(s)=w130:i32)
        n103 = Greater Or Equal?(x=w130, y=2) -> (x >= y?=w128:bool)
        n104 = case shown="True" w128 {
          frame False {
          }
          frame True {
            n105 = property on="Calculate\nTrajectory" class="Bool (strict)"("Val(Sgnl)"=TRUE ("Value (Signaling)")) -> ()  [unwired: 2 in, 2 out]
          }
        }
      }
      event "End Program": Value Change {
        n106 = event-data() -> ("NewVal"=w140:bool)  [unwired: 1 in, 5 out]
        n107 = case shown="True" w140 {
          frame False {
          }
          frame True {
            # "The code doesn't seem to work\ninside the event handler...."
            n108 = local write "Terminate"(TRUE ("Terminate")) -> ()
          }
        }
      }
      event "WriteJSONFile": Value Change {
        n109 = event-data() -> ("NewVal"=w142:bool)  [unwired: 1 in, 5 out]
        n110 = local read "Trajectory\nCompleted\nError Free"() -> (w144:bool)
        n111 = And(x=w142, y=w144) -> (x .and. y?=w143:bool)
        n112 = case shown="True" w143 {
          frame False {
          }
          frame True {
            n113 = local read "Trajectory Type"() -> (w154:enum32{"Radio Selection 1", "Radio Selection 2"})
            n114 = local read "TRAJECTORY"() -> (w155:T7)
            n115 = case shown="\"Radio Selection 1\", Default" w154 {
              tunnel: w155 -> [w160 w162]
              tunnel: [w159 w162] -> w152
              tunnel: [TRUE FALSE] -> _
              frame "Radio Selection 1", Default {
                # "Relative"
                n116 = call <vilib>:"Util_Trajectory_Absolute_To_Relative.vi"("absTRAJECTORY"=w160) -> ("outputRelativeTRAJECTORY"=w159:T7)  [unwired: 10 in]
              }
              frame "Radio Selection 2" {
                # "Absolute"
              }
            }
            n117 = call <vilib>:"Trajectory_GetStates.vi"("TRAJECTORY"=w152) -> ("States"=w153:T8[])  [unwired: 10 in]
            n118 = call "Create_Trajectory_Traj_Meters_To_PW_Units.vi"("States in_M"=w153, "PathWeaver Length Units"="PathWeaver Length Units") -> ("States out_UNITS"=w151:T8[])  [unwired: 9 in]
            n119 = call <vilib>:"Trajectory_New.vi"("TRAJ_STATES"=w151) -> ("TRAJECTORY"=w150:T7)  [unwired: 10 in]
            n120 = Path To String(path="Trajectory JSON File Name") -> (string=w147:string)
            n121 = call <vilib>:"TrajectoryUtil_toPathWeaverJSON.vi"("inTRAJECTORY"=w150, "FileName"=w147) -> ("error out"=w146:errorcluster)  [unwired: 8 in, 1 out]
            "Write CSV File Error" <- w146
            n122 = case shown="Error .." w146 {
              tunnel: [TRUE ("File Saved\nWithout\nError") FALSE ("File Saved\nWithout\nError")] -> w145
              frame No Error {
              }
              frame Error {
              }
            }
            "JSON File Saved\nWithout Error" <- w145
          }
        }
      }
      event "ReadConfigFile": Value Change {
        n123 = event-data() -> ("NewVal"=w163:bool)  [unwired: 1 in, 5 out]
        n124 = case shown="True" w163 {
          frame False {
          }
          frame True {
            # "#TODO Fix read file for\nV5 variant issue."
            # "#TODO Need to clear and rebuild cursors!!!"
            # "Read\nFile"
            # "Read config from trajectory File"
            n125 = call-poly <vilib>:"Read From XML File.vi"("XML File Path"="Read Config File Name") -> ("error out"=w166:errorcluster, "XML Elements"=w165:string)  [unwired: 8 in, 1 out]
            n126 = case shown="No Error" w166 {
              tunnel: w165 -> [w173 _]
              tunnel: w166 -> [w172 w289]
              tunnel: [w176 w289] -> w167
              tunnel: [w175 FALSE] -> w168
              tunnel: [w177 "" ("Write Config File Comment")] -> w169
              frame No Error {
                # "parse\nXML"
                # "A little bit of a \nkludge to read \nboth v2 and v1\nfile formats...."
                n127 = local read "Units Selector"() -> (w170:T12)
                n128 = call "Create_Trajectory_Config_Parse_V1_V2_V3.vi"("error in (no error)"=w172, "Units Selector"=w170, "XML Elements"=w173) -> ("error out"=w174:errorcluster, "TrajCreateConfig"=w171:T20)  [unwired: 7 in]
                n129 = case shown="No Error" w174 {
                  tunnel: w171 -> [w185 _]
                  tunnel: [w183 "" ("Write Config File Comment")] -> w177
                  tunnel: w174 -> [w182 w285]
                  tunnel: [w181 w285] -> w176
                  tunnel: [w184 FALSE] -> w175
                  frame No Error {
                    # "Create and draw \ntrajectory."
                    n130 = flat-sequence {
                      tunnel: w185 -> [w200]
                      tunnel: [TRUE] -> w184
                      tunnel: [w257] -> w183
                      tunnel: w182 -> [w203]
                      tunnel: [w203] -> w181
                      tunnel: [w201] -> w180
                      frame #0 {
                        # "Update cursors..."
                        # "Field is always\ninches..."
                        # "Write to local\nuser controls"
                        # "not used"
                        # "not used"
                        n131 = Unbundle By Name(w200) -> ("Write Config File Name"=w216:path, "Write Config File Comment"=w257:string, "WayPoints"=w208:T6[], "TRAJECTORY_CONFIG"=w192:T5, "IsCubic"=w211:bool, "Units Selector"=w205:T12, "UseWeights"=w214:bool)
                        n132 = Unbundle By Name(w200) -> ("FieldName"=w199:string)
                        n133 = Unbundle By Name(w192) -> ("MaxVelocity"=w265:dbl, "Max Acceleration"=w264:dbl, "Reversed"=w263:bool)  [unwired: 2 out]
                        n134 = call <vilib>:"TrajectoryConfig_GetKinematicsDiffDriveContraint.vi"("inTRAJECTORY_CONFIG"=w192) -> ("Constraint Exists"=w195:bool, "Diff Drive Kinematics Constraint"=w188:T21)  [unwired: 9 in]
                        n135 = call <vilib>:"TrajectoryConfig_GetCentripetalAccelConstraint.vi"("inTRAJECTORY_CONFIG"=w192) -> ("Constraint Exists"=w194:bool, "Centripital Accleration Constraint"=w198:T23)  [unwired: 9 in]
                        n136 = call <vilib>:"TrajectoryConfig_GetVoltageDiffDriveConstraint.vi"("inTRAJECTORY_CONFIG"=w192) -> ("Constraint Exists"=w193:bool, "Differential Drive Voltage Constraint"=w197:T24)  [unwired: 9 in]
                        n137 = call <vilib>:"TrajectoryConfig_GetKinematicsMecanumDriveConstraint.vi"("inTRAJECTORY_CONFIG"=w192) -> ("Constraint Exists"=w190:bool, "Mecanum Drive Kinematics Constraint"=w196:T25)  [unwired: 9 in]
                        n138 = Unbundle By Name(w196) -> ("MECA_DRIVE_KINEMATICS.FrontLeft"=w233:T2, "MECA_DRIVE_KINEMATICS.FrontRight"=w234:T2, "MECA_DRIVE_KINEMATICS.RearLeft"=w235:T2, "MECA_DRIVE_KINEMATICS.RearRight"=w236:T2)
                        n139 = call <vilib>:"TrajectoryConfig_GetKinematicsSwerveDriveConstraint.vi"("inTRAJECTORY_CONFIG"=w192) -> ("Constraint Exists"=w189:bool, "Swerver Drive Kinematics Constraint"=w191:T28)  [unwired: 9 in]
                        n140 = Unbundle By Name(w188) -> ("DIFF_DRIVE_KINEMATICS.TrackWidth_Meters"=w261:dbl)
                        n141 = Unbundle By Name(w198) -> ("Max Cent Accel"=w259:dbl)
                        n142 = Unbundle By Name(w197) -> ("Max Voltage"=w258:dbl, "SIMPLE_MOTOR_FF"=w219:T13)
                        n143 = Unbundle By Name(w191) -> ("SwerveKinematics.Modules"=w253:T2[])
                        n144 = property on="Field Selector" class="CmbBox"("Val(Sgnl)"=w199) -> ()  [unwired: 2 in, 2 out]
                        n145 = Unbundle By Name(w219) -> ("Ks"=w228:dbl, "Kv"=w227:dbl, "Ka"=w220:dbl)
                        n146 = call "Create_Trajectory_All_WP_Meters_To_Units.vi"("Units Selector"=TrajCreateUnitsENUM."Inches", "WayPoints_M"=w208) -> ("outWayPoints_UNITS"=w207:T6[])  [unwired: 9 in]
                        n147 = call "Create_Trajectory_All_WP_Meters_To_Units.vi"("Units Selector"=w205, "WayPoints_M"=w208) -> ("outWayPoints_UNITS"=w202:T6[])  [unwired: 9 in]
                        n148 = case shown="True" w211 {
                          tunnel: [enum32{"Radio Selection 1", "Radio Selection 2"}."Radio Selection 2" ("Spline Type") enum32{"Radio Selection 1", "Radio Selection 2"}."Radio Selection 1" ("Spline Type")] -> w268
                          frame False {
                          }
                          frame True {
                          }
                        }
                        n149 = Reciprocal(x=w227) -> (1/x=w226:dbl)
                        n150 = Reciprocal(x=w220) -> (1/x=w223:dbl)
                        n151 = call "ChangeFileExtension.vi"("NewExtenion"=".json", "In FileName"=w216) -> ("Out FileName"=w215:path)  [unwired: 9 in]
                        n152 = call "ChangeFileExtension.vi"("NewExtenion"=".csv", "In FileName"=w216) -> ("Out FileName"=w256:path)  [unwired: 9 in]
                        n153 = call <vilib>:"Translation2d_GetXY.vi"("In Translation"=w233) -> ("Y"=w250:dbl, "X"=w252:dbl)  [unwired: 9 in]
                        n154 = call <vilib>:"Translation2d_GetXY.vi"("In Translation"=w234) -> ("Y"=w246:dbl, "X"=w248:dbl)  [unwired: 9 in]
                        n155 = call <vilib>:"Translation2d_GetXY.vi"("In Translation"=w235) -> ("Y"=w242:dbl, "X"=w244:dbl)  [unwired: 9 in]
                        n156 = for {
                          tunnel: w253 -> [w277] mode=indexing
                          tunnel: [w276] -> w254 mode=indexing
                          tunnel: w205 -> [w275]
                          n157 = call <vilib>:"Translation2d_GetXY.vi"("In Translation"=w277) -> ("Y"=w279:dbl, "X"=w281:dbl)  [unwired: 9 in]
                          n158 = call "Create_Trajectory_Value_Meters_To_Units.vi"("Units Selector"=w275, "Meters"=w281) -> ("Units"=w280:dbl)  [unwired: 9 in]
                          n159 = call "Create_Trajectory_Value_Meters_To_Units.vi"("Units Selector"=w275, "Meters"=w279) -> ("Units"=w278:dbl)  [unwired: 9 in]
                          n160 = call <vilib>:"Translation2d_Create.vi"("Y"=w278, "X"=w280) -> ("TRANSLATION"=w276:T2)  [unwired: 9 in]
                        }
                        n161 = call <vilib>:"Translation2d_GetXY.vi"("In Translation"=w236) -> ("Y"=w238:dbl, "X"=w240:dbl)  [unwired: 9 in]
                        n162 = call "Create_Trajectory_Value_Meters_To_Units.vi"("Units Selector"=w205, "Meters"=w226) -> ("Units"=w225:dbl)  [unwired: 9 in]
                        n163 = local write "WayPoints"(w202) -> ()
                        n164 = for {
                          tunnel: w207 -> [w273] mode=indexing
                          tunnel: [w270] -> w204 mode=indexing
                          n165 = Unbundle By Name(w273) -> ("X"=w272:dbl, "Y"=w271:dbl)
                          n166 = Bundle By Name(cluster=T19 {"Name"="Cursor", "Color"=915580, "Style"=4, "Point Style"=2, "Name Visible"=FALSE, "Allow Drag"=TRUE, "Cursor Mode"=0, "Plot"=0, "Index"=0, "Position"={"X"=315.0, "Y"=162.0}, "X Scale"=0, "Y Scale"=0, "Watch Plots"=[], "Watch All Plots"=FALSE, "Plot Area"=0, "Label Offset"={"X"=0.0, "Y"=0.0}} ("new element/subarray"), "Position.X"=w272, "Position.Y"=w271) -> (w270:T19)
                        }
                        n167 = call "Create_Trajectory_Value_Meters_To_Units.vi"("Units Selector"=w205, "Meters"=w223) -> ("Units"=w222:dbl)  [unwired: 9 in]
                        n168 = local write "outTRAJECTORY_CONFIG"(w192) -> ()
                        n169 = local write "Units Selector"(w205) -> ()
                        n170 = local write "WayPoints_M"(w208) -> ()
                        n171 = local write "Trajectory JSON File Name"(w215) -> ()
                        n172 = local write "Trajectory CSV File Name"(w256) -> ()
                        n173 = call "Create_Trajectory_Value_Meters_To_Units.vi"("Units Selector"=w205, "Meters"=w252) -> ("Units"=w251:dbl)  [unwired: 9 in]
                        n174 = call "Create_Trajectory_Value_Meters_To_Units.vi"("Units Selector"=w205, "Meters"=w265) -> ("Units"=w266:dbl)  [unwired: 9 in]
                        n175 = call "Create_Trajectory_Value_Meters_To_Units.vi"("Units Selector"=w205, "Meters"=w264) -> ("Units"=w267:dbl)  [unwired: 9 in]
                        n176 = call "Create_Trajectory_Value_Meters_To_Units.vi"("Units Selector"=w205, "Meters"=w248) -> ("Units"=w247:dbl)  [unwired: 9 in]
                        n177 = local write "IsCubic"(w211) -> ()
                        n178 = local write "UseWeights"(w214) -> ()
                        n179 = local write "Write Config File Name"(w216) -> ()
                        n180 = local write "Write Config File Comment"(w257) -> ()
                        n181 = local write "Trajectory File Comment"(w257) -> ()
                        n182 = call "Create_Trajectory_Value_Meters_To_Units.vi"("Units Selector"=w205, "Meters"=w244) -> ("Units"=w243:dbl)  [unwired: 9 in]
                        n183 = Reciprocal(x=w225) -> (1/x=w224:dbl)
                        n184 = call "Create_Trajectory_Value_Meters_To_Units.vi"("Units Selector"=w205, "Meters"=w240) -> ("Units"=w239:dbl)  [unwired: 9 in]
                        n185 = Reciprocal(x=w222) -> (1/x=w221:dbl)
                        n186 = call "Create_Trajectory_Value_Meters_To_Units.vi"("Units Selector"=w205, "Meters"=w250) -> ("Units"=w249:dbl)  [unwired: 9 in]
                        n187 = call "Create_Trajectory_Value_Meters_To_Units.vi"("Units Selector"=w205, "Meters"=w246) -> ("Units"=w245:dbl)  [unwired: 9 in]
                        n188 = Array Size(array=w202) -> (size(s)=w201:i32)
                        n189 = local write "Use Mecanum \nDrive Kinematics\nConstraint"(w190) -> ()
                        n190 = call "Create_Trajectory_Value_Meters_To_Units.vi"("Units Selector"=w205, "Meters"=w242) -> ("Units"=w241:dbl)  [unwired: 9 in]
                        n191 = call "Create_Trajectory_Value_Meters_To_Units.vi"("Units Selector"=w205, "Meters"=w238) -> ("Units"=w237:dbl)  [unwired: 9 in]
                        n192 = call "Create_Trajectory_Value_Meters_To_Units.vi"("Units Selector"=w205, "Meters"=w261) -> ("Units"=w262:dbl)  [unwired: 9 in]
                        n193 = call "Create_Trajectory_Value_Meters_To_Units.vi"("Units Selector"=w205, "Meters"=w259) -> ("Units"=w260:dbl)  [unwired: 9 in]
                        n194 = local write "Use Swerve Drive\nKinematics\nConstraint"(w189) -> ()
                        n195 = local write "Use Centripetal\nAcceleration\nConstaint"(w194) -> ()
                        n196 = call <vilib>:"SimpleMotorFF_New.vi"("Ka"=w221, "Kv"=w224, "Ks"=w228) -> ("SIMPLE_MOTOR_FF"=w218:T13)  [unwired: 8 in]
                        n197 = local write "Use Diff Drive\nKinematic\nConstraint"(w195) -> ()
                        n198 = local write "MaxVelocity"(w266) -> ()
                        n199 = local write "MaxAcceleration"(w267) -> ()
                        n200 = local write "Spline Type"(w268) -> ()
                        n201 = call <vilib>:"Translation2d_Create.vi"("Y"=w249, "X"=w251) -> ("TRANSLATION"=w232:T2)  [unwired: 9 in]
                        n202 = local write "Reverse"(w263) -> ()
                        n203 = local write "Use Diff Drive\nVoltage\nConstraint"(w193) -> ()
                        n204 = call <vilib>:"Translation2d_Create.vi"("Y"=w245, "X"=w247) -> ("TRANSLATION"=w231:T2)  [unwired: 9 in]
                        n205 = local write "CSV File Saved\nWithout Error"(FALSE ("File Saved\nWithout\nError")) -> ()
                        n206 = local write "Trajectory\nCompleted\nError Free"(FALSE ("Trajectory\nCompleted\nError Free")) -> ()
                        n207 = local write "Config File Saved\nWithout Error"(FALSE ("File Saved\nWithout\nError")) -> ()
                        n208 = local write "JSON File Saved\nWithout Error"(FALSE ("File Saved\nWithout\nError")) -> ()
                        n209 = call <vilib>:"Translation2d_Create.vi"("Y"=w241, "X"=w243) -> ("TRANSLATION"=w230:T2)  [unwired: 9 in]
                        n210 = call <vilib>:"Translation2d_Create.vi"("Y"=w237, "X"=w239) -> ("TRANSLATION"=w229:T2)  [unwired: 9 in]
                        n211 = local write "Max Cent Accel"(w260) -> ()
                        n212 = local write "Track Width"(w262) -> ()
                        n213 = local write "SIMPLE_MOTOR_FF"(w218) -> ()
                        n214 = local write "Max Voltage"(w258) -> ()
                        n215 = local write "Left Front"(w232) -> ()
                        n216 = local write "Right Front"(w231) -> ()
                        n217 = local write "Right Rear"(w229) -> ()
                        n218 = local write "Left Rear"(w230) -> ()
                        n219 = local write "Wheels"(w254) -> ()
                        n220 = property on="Position" class="XYGraph (strict)"("CrsrList"=w204) -> ()  [unwired: 2 in, 2 out]
                      }
                    }
                    n221 = Greater Or Equal?(x=w180, y=2) -> (x >= y?=w178:bool)
                    n222 = case shown="True" w178 {
                      frame False {
                        n223 = local write "TRAJECTORY"(T7 {"TotalTImeSecs"=0.0, "States"=[]} ("TRAJECTORY")) -> ()
                      }
                      frame True {
                        n224 = property on="Calculate\nTrajectory" class="Bool (strict)"("Val(Sgnl)"=TRUE ("Value (Signaling)")) -> ()  [unwired: 2 in, 2 out]
                      }
                    }
                  }
                  frame Error {
                  }
                }
              }
              frame Error {
              }
            }
            "Config File Read\nWithout Error" <- w168
            "Config File  Read Error" <- w167
            "Read Config File Comment" <- w169
          }
        }
      }
      event "WriteConfigFile": Value Change {
        n225 = event-data() -> ("NewVal"=w291:bool)  [unwired: 1 in, 5 out]
        n226 = local read "Trajectory\nCompleted\nError Free"() -> (w292:bool)
        n227 = And(x=w291, y=w292) -> (x .and. y?=w290:bool)
        n228 = case shown="True" w290 {
          frame False {
          }
          frame True {
            # "Convert\ninternal\nto V4"
            # "write xml\nfile"
            # "convert\nto xml\nstring"
            n229 = local read "outTRAJECTORY_CONFIG"() -> (w298:T5)
            n230 = local read "Field Selector"() -> (w306:string)
            n231 = local read "WayPoints_M"() -> (w314:T6[])
            n232 = local read "UseWeights"() -> (w315:bool)
            n233 = local read "IsCubic"() -> (w317:bool)
            n234 = local read "Units Selector"() -> (w316:T12)
            n235 = Unbundle By Name(w298) -> ("Constraints"=w297:variant[])
            n236 = Index Array(array=w297) -> (element #3=w295:variant)  [unwired: 3 in, 2 out]
            n237 = Bundle By Name(cluster=T20 {"Write Config File Name"=path "", "Write Config File Comment"="", "WayPoints"=[], "TRAJECTORY_CONFIG"={"MaxVelocity"=0.0, "Max Acceleration"=0.0, "StartVelocity"=0.0, "End Velocity"=0.0, "Reversed"=FALSE, "Constraints"=[]}, "IsCubic"=FALSE, "Units Selector"=enum."Inches", "UseWeights"=FALSE, "FieldName"=""} ("TrajCreateConfig"), "Write Config File Name"="Write Config File Name", "Write Config File Comment"="Write Config File Comment", "WayPoints"=w314, "TRAJECTORY_CONFIG"=w298, "IsCubic"=w317, "Units Selector"=w316, "UseWeights"=w315, "FieldName"=w306) -> (w305:T20)
            n238 = Variant To Data(type=T1 {"BottomLeftPoint"={"X"=0.0, "Y"=0.0}, "TopRightPoint"={"X"=0.0, "Y"=0.0}, "Constraint"=variant, "Constraint Type"=enum."DIFF DRIVE KINEMATICS"} ("RECT_REGION_CONSTRAINT"), Variant=w295) -> (data=w294:T1)  [unwired: 1 in, 1 out]
            n239 = Flatten To XML(anything=w294) -> (xml string=w303:string)
            "xml string" <- w303
            n240 = local write "Trajectory File Comment"("Write Config File Comment") -> ()
            n241 = call <vilib>:"Easy Generate XML__JKI EasyXML.vi"("LabVIEW Data"=w294) -> ("XML String"=w301:string)  [unwired: 9 in, 1 out]
            n242 = Unflatten From XML(xml string=w303, type=w294) -> (value=→"value":T1, error out=→"error out":errorcluster)  [unwired: 1 in]
            n243 = call "Creat_Traj_Config_Convert_V_internal_To_V4.vi"("TrajCreateConfig V_Internal"=w305) -> ("TrajCreateConfig V4"=w304:T31)  [unwired: 10 in]
            n244 = call <vilib>:"Easy Parse XML__JKI EasyXML.vi"("LabVIEW Data (Type)"=w294, "XML String"=w301) -> ("error out"=→"error out 2":errorcluster, "LabVIEW Data"=→"LabVIEW Data":variant)  [unwired: 8 in]
            n245 = Flatten To XML(anything=w304) -> (xml string=w311:string)
            n246 = call-poly <vilib>:"Write to XML File.vi"("Standalone? (T)"=TRUE, "XML Input"=w311, "XML File Path"="Write Config File Name") -> ("error out"=w312:errorcluster)  [unwired: 6 in, 2 out]
            "Write Config FIle Error" <- w312
            n247 = case shown="No Error" w312 {
              tunnel: [TRUE ("File Saved\nWithout\nError") FALSE ("File Saved\nWithout\nError")] -> w307
              frame No Error {
              }
              frame Error {
              }
            }
            "Config File Saved\nWithout Error" <- w307
          }
        }
      }
      event "WriteTrajFile": Value Change {
        n248 = event-data() -> ("NewVal"=w321:bool)  [unwired: 1 in, 5 out]
        n249 = local read "Trajectory\nCompleted\nError Free"() -> (w322:bool)
        n250 = And(x=w321, y=w322) -> (x .and. y?=w320:bool)
        n251 = case shown="True" w320 {
          frame False {
          }
          frame True {
            n252 = local read "UseWeights"() -> (w333:bool)
            n253 = local read "outTRAJECTORY_CONFIG"() -> (w332:T5)
            n254 = local read "TRAJECTORY"() -> (w331:T7)
            n255 = local read "WayPoints_M"() -> (w330:T6[])
            n256 = local read "IsCubic"() -> (w334:bool)
            n257 = case shown="\"Radio Selection 1\", Default" "Trajectory Type" {
              tunnel: w331 -> [w339 w341]
              tunnel: [w338 w341] -> w325
              tunnel: [TRUE FALSE] -> w327
              frame "Radio Selection 1", Default {
                # "Relative"
                n258 = call <vilib>:"Util_Trajectory_Absolute_To_Relative.vi"("absTRAJECTORY"=w339) -> ("outputRelativeTRAJECTORY"=w338:T7)  [unwired: 10 in]
              }
              frame "Radio Selection 2" {
                # "Absolute"
              }
            }
            n259 = call <vilib>:"Util_Trajectory_WriteFile.vi"("Trajectory is Cubic"=w334, "UseWeights"=w333, "Trajectory Is Relative"=w327, "TRAJECTORY_CONFIG"=w332, "UtilityWayPoints"=w330, "TRAJECTORY"=w325, "Comment"="Trajectory File Comment", "Trajectory File Name"="Trajectory CSV File Name") -> ("error out"=w326:errorcluster)  [unwired: 3 in]
            "Write Trajectory\nFile Error" <- w326
            n260 = local write "Write Config File Comment"("Trajectory File Comment") -> ()
            n261 = case shown="Error .." w326 {
              tunnel: [TRUE ("File Saved\nWithout\nError") FALSE ("File Saved\nWithout\nError")] -> w323
              frame No Error {
              }
              frame Error {
              }
            }
            "CSV File Saved\nWithout Error" <- w323
          }
        }
      }
      event "Field Selector": Value Change {
        n262 = event-data() -> ("NewVal"=w343:string)  [unwired: 1 in, 5 out]
        n263 = local read "FIeldSelectorHasItems"() -> (w342:bool)
        n264 = case shown="True" w342 {
          tunnel: w343 -> [_ w351]
          frame False {
          }
          frame True {
            n265 = local read "FIeld Image"() -> (w344:T4)
            n266 = call "Create_Trajectory_Get_Field_Info.vi"("Field Selector"=w351) -> ("File"=w352:string, "input cluster"=w350:T16)  [unwired: 9 in]
            n267 = call "Create_Trajectory_Read_Field_Pic.vi"("file name"=w352) -> ("Image Error"=w345:errorcluster, "Image Data"=w349:T4)  [unwired: 7 in, 2 out]
            n268 = case shown="Error .." w345 {
              frame Error {
                n269 = One Button Dialog(message="The field_picture file could not be read.  Execution will continue normally with a blank playing field.") -> ()  [unwired: 1 in, 1 out]
              }
              frame No Error {
              }
            }
            n270 = call "Create_Trajectory_Field_Crop_and_Scale.vi"("Disp Y Size Pixel"=430, "Disp X Size Pixel"=860, "Field Image"=w349, "field Info"=w350, "Display Image"=w344) -> ("Disp Image Out"=→"Field Display":T4)  [unwired: 5 in, 1 out]
          }
        }
      }
      event "Calculate\nTrajectory": Value Change {
        n271 = event-data() -> ("NewVal"=w354:bool)  [unwired: 1 in, 5 out]
        n272 = case shown="True" w354 {
          frame False {
          }
          frame True {
            w366 = FALSE ("File Saved\nWithout\nError")
            # "Turn it off...."
            # "FIELD POSITION\nGRAPH"
            # "Inches/Sec"
            # "Inches"
            # "in meters"
            # "construct the trajectory\nconfiguration information"
            # "trajectory \nmeters, radians"
            n273 = local read "Use Diff Drive\nKinematic\nConstraint"() -> (w392:bool)
            n274 = local read "MaxAcceleration M/S^2"() -> (w394:dbl)
            n275 = local read "Use Rectangular Region\nDiff Drive Kinematics\nConstraint"() -> (w362:bool)
            n276 = local read "Use Swerve Drive\nKinematics\nConstraint"() -> (w397:bool)
            n277 = local read "MaxVelocity M/S"() -> (w395:dbl)
            n278 = local read "Rect Reg Top Right M"() -> (w358:T2)
            n279 = local read "Max Accel M/Sec^2"() -> (w356:dbl)
            n280 = local read "Rect Reg Bot Left M"() -> (w359:T2)
            n281 = local read "Max Sped M/Sec"() -> (w357:dbl)
            n282 = local read "Track Width M"() -> (w355:dbl)
            n283 = local read "Track Width M"() -> (w396:dbl)
            n284 = local read "Wheels M"() -> (w398:T2[])
            n285 = local read "Reverse"() -> (w393:bool)
            n286 = call <vilib>:"TrajectoryConfig_Create.vi"("MaxAcceleration"=w394, "MaxVelocity"=w395) -> ("TRAJECTORY_CONFIG"=w378:T5)  [unwired: 9 in]
            n287 = local read "WayPoints_M"() -> (w383:T6[])
            n288 = local read "UseWeights"() -> (w384:bool)
            n289 = call <vilib>:"TrajectoryConfig_setReversed.vi"("Reversed"=w393, "inTRAJECTORY_CONFIG"=w378) -> ("outTRAJECTORY_CONFIG"=w379:T5)  [unwired: 9 in]
            n290 = call <vilib>:"DiffKinematics_New.vi"("TrackWidth_Meters"=w396) -> ("DIFF_DRIVE_KINEMATICS"=w391:T22)  [unwired: 10 in]
            n291 = local read "Use Centripetal\nAcceleration\nConstaint"() -> (w389:bool)
            n292 = local read "Max Cent Accel M/S^2"() -> (w390:dbl)
            n293 = local read "Use Diff Drive\nVoltage\nConstraint"() -> (w386:bool)
            n294 = local read "Use Mecanum \nDrive Kinematics\nConstraint"() -> (w399:bool)
            n295 = case shown="True" w392 {
              tunnel: w379 -> [w438 w441]
              tunnel: [w438 w440] -> w368
              tunnel: w391 -> [_ w439]
              frame False {
              }
              frame True {
                n296 = call <vilib>:"TrajectoryConfig_setKinematicsDiffDrive.vi"("DIFF_DRIVE_KINEMATICS"=w439, "inTRAJECTORY_CONFIG"=w441) -> ("outTRAJECTORY_CONFIG"=w440:T5)  [unwired: 9 in]
              }
            }
            n297 = local read "Left Front M"() -> (w400:T2)
            n298 = local read "Right Front M"() -> (w401:T2)
            n299 = local read "Left Rear M"() -> (w402:T2)
            n300 = local read "Right Rear M"() -> (w403:T2)
            n301 = case shown="True" w389 {
              tunnel: w368 -> [w434 w437]
              tunnel: [w434 w436] -> w370
              tunnel: w390 -> [_ w435]
              frame False {
              }
              frame True {
                n302 = call <vilib>:"TrajectoryConfig_setCentripetalAccel.vi"("Max Cent Accel"=w435, "inTRAJECTORY_CONFIG"=w437) -> ("outTRAJECTORY_CONFIG"=w436:T5)  [unwired: 9 in]
              }
            }
            n303 = local read "SIMPLE_MOTOR_FF M"() -> (w388:T13)
            n304 = local read "Max Voltage"() -> (w387:dbl)
            n305 = case shown="True" w386 {
              tunnel: w370 -> [w428 w433]
              tunnel: [w428 w432] -> w371
              tunnel: w387 -> [_ w431]
              tunnel: w388 -> [_ w430]
              tunnel: w391 -> [_ w429]
              frame False {
              }
              frame True {
                n306 = call <vilib>:"TrajectoryConfig_setVoltageDiffDrive.vi"("SIMPLE_MOTOR_FF"=w430, "DIFF_DRIVE_KINEMATICS"=w429, "Max Voltage"=w431, "inTRAJECTORY_CONFIG"=w433) -> ("outTRAJECTORY_CONFIG"=w432:T5)  [unwired: 7 in]
              }
            }
            n307 = case shown="True" w397 {
              tunnel: [w423 w427] -> w373
              tunnel: w371 -> [w423 w426]
              tunnel: w398 -> [_ w424]
              frame False {
              }
              frame True {
                n308 = call <vilib>:"SwerveKinematics_NewX.vi"("Wheels"=w424) -> ("SWERVE_DRIVE_KINEMATICS"=w425:T29)  [unwired: 10 in]
                n309 = call <vilib>:"TrajectoryConfig_setKinematicsSwerveDrive.vi"("SWERVE_DRIVE_KINEMATICS"=w425, "inTRAJECTORY_CONFIG"=w426) -> ("outTRAJECTORY_CONFIG"=w427:T5)  [unwired: 9 in]
              }
            }
            n310 = case shown="True" w399 {
              tunnel: [w415 w422] -> w361
              tunnel: w373 -> [w415 w421]
              tunnel: w400 -> [_ w419]
              tunnel: w401 -> [_ w418]
              tunnel: w402 -> [_ w417]
              tunnel: w403 -> [_ w416]
              frame False {
              }
              frame True {
                n311 = call <vilib>:"MecaKinematics_New.vi"("RearRight"=w416, "RearLeft"=w417, "FrontRight"=w418, "FrontLeft"=w419) -> ("MECA_DRIVE_KINEMATICS"=w420:T26)  [unwired: 7 in]
                n312 = call <vilib>:"TrajectoryConfig_setKinematicsMecanumDrive.vi"("MECA_DRIVE_KINEMATICS"=w420, "inTRAJECTORY_CONFIG"=w421) -> ("outTRAJECTORY_CONFIG"=w422:T5)  [unwired: 9 in]
              }
            }
            n313 = case shown="True" w362 {
              tunnel: w361 -> [w404 w411]
              tunnel: [w404 w410] -> w360
              tunnel: w359 -> [_ w409]
              tunnel: w358 -> [_ w408]
              tunnel: w357 -> [_ w407]
              tunnel: w356 -> [_ w406]
              tunnel: w355 -> [_ w405]
              frame False {
              }
              frame True {
                n314 = call <vilib>:"DiffKinematics_New.vi"("TrackWidth_Meters"=w405) -> ("DIFF_DRIVE_KINEMATICS"=w413:T22)  [unwired: 10 in]
                n315 = call <vilib>:"DiffDriveKinematicsConstraint_New.vi"("DIFF_DRIVE_KINEMATICS"=w413, "Max Accel (M/S2)"=w406, "Max Speed (M/S)"=w407) -> ("DIFF_DRIVE_KINE_CONSTRAINT"=w414:T21)  [unwired: 8 in]
                n316 = call <vilib>:"RectRegionConstraint_New.vi"("Constraint Data Cluster"=w414, "TopRightPoint"=w408, "BottomLeftPoint"=w409) -> ("RECT_REGION_CONSTRAINT"=w412:T1)  [unwired: 8 in]
                n317 = call <vilib>:"TrajectoryConfig_AddConstraint.vi"("Constraint"=w412, "inTRAJECTORY_CONFIG"=w411) -> ("outTRAJECTORY_CONFIG"=w410:T5)  [unwired: 9 in]
              }
            }
            "outTRAJECTORY_CONFIG" <- w360
            n318 = call "Create_Trajectory_Make_Trajectory.vi"("TRAJECTORY_CONFIG"=w360, "Spline Type"="Spline Type", "WayPoints"=w383, "UseWeights"=w384) -> ("error out"=→"Trajectory calculation error":errorcluster, "Is Cubic"=w385:bool, "TRAJECTORY"=w365:T7)  [unwired: 5 in]
            "TRAJECTORY" <- w365
            n319 = local write "IsCubic"(w385) -> ()
            n320 = call <vilib>:"Trajectory_GetStates.vi"("TRAJECTORY"=w365) -> ("States"=w381:T8[])  [unwired: 10 in]
            "Trajectory States" <- w381
            n321 = call "Create_Trajectory_Prepare_Graph.vi"("TRAJECTORY"=w365) -> ("Array"=→"Trajectory Data":cluster{dbl[], dbl[]}[])  [unwired: 10 in]
            n322 = call "Create_Trajectory_Build_Trajectory_Field_Plot.vi"("TrackWidth_Meters"=w396, "WayPoints"=w383, "States"=w381) -> ("Array"=→"Position":cluster{dbl[], dbl[]}[])  [unwired: 8 in]
            n323 = call "Create_Trajectory_Check_Diff_Drive_Max_Speed.vi"("Use Diff Drive\nKinematic\nConstraint"=w392, "Max Speed M/S"=w395, "DIFF_DRIVE_KINEMATICS"=w391, "States"=w381) -> ("Inches/Second"=→"differential \ndrive \nmax speed":dbl, "Max Speed Exceeded"=w382:bool)  [unwired: 6 in]
            n324 = Array Size(array=w381) -> (size(s)=w375:i32)
            "Traj States\nSize" <- w375
            n325 = Not(x=w382) -> (.not. x?=w377:bool)
            n326 = Greater Than 0?(x=w375) -> (x > 0?=w376:bool)
            n327 = And(x=w376, y=w377) -> (x .and. y?=→"Trajectory\nCompleted\nError Free":bool)
            n328 = local write "Config File Saved\nWithout Error"(w366) -> ()
            n329 = local write "JSON File Saved\nWithout Error"(w366) -> ()
            n330 = local write "CSV File Saved\nWithout Error"(w366) -> ()
            n331 = local write "Calculate\nTrajectory"(FALSE ("Calculate\nTrajectory")) -> ()
          }
        }
      }
      event "Position": Cursor Grab {
        # "Remember which one is selected"
        # "Grab a waypoint"
        n332 = event-data() -> ("CursIdx"=w442:i32)  [unwired: 1 in, 8 out]
        n333 = local write "Index"(w442) -> ()
      }
      event "Position": Cursor Release {
        # "If there are 2 or more waypoints, recalc the trajectory..."
        # "Don't forget the last selected cursor.."
        n334 = event-data() -> ()  [unwired: 1 in, 9 out]
        n335 = disable-structure shown="Disabled" {
          frame Disabled {
            n336 = local write "Index"(-1 ("Index")) -> ()
          }
          frame Enabled {
          }
        }
        n337 = local read "Units Selector"() -> (w444:T12)
        n338 = local read "WayPoints"() -> (w445:T6[])
        n339 = call "Create_Trajectory_All_WP_Units_To_Meters.vi"("Units Selector"=w444, "WayPoints"=w445) -> ("Array"=w443:T6[])  [unwired: 9 in]
        n340 = Array Size(array=w443) -> (size(s)=w446:i32)
        n341 = local write "WayPoints_M"(w443) -> ()
        n342 = Greater Or Equal?(x=w446, y=2) -> (x >= y?=w447:bool)
        n343 = case shown="True" w447 {
          frame False {
          }
          frame True {
            n344 = property on="Calculate\nTrajectory" class="Bool (strict)"("Val(Sgnl)"=TRUE ("Value (Signaling)")) -> ()  [unwired: 2 in, 2 out]
          }
        }
      }
      event "Position": Cursor Move {
        # "#NOTE Probably can use CursIdx here.   We keep our own index so that we can still change the last selected item even if it isn't selected any more."
        n345 = event-data() -> ("CursLoc"=w451:cluster{"X":dbl, "Y":dbl})  [unwired: 1 in, 8 out]
        n346 = local read "Index"() -> (w453:i32)
        n347 = Greater Or Equal To 0?(x=w453) -> (x >= 0?=w452:bool)
        n348 = case shown="True" w452 {
          tunnel: w453 -> [w464 _]
          tunnel: w451 -> [w462 _]
          frame True {
            n349 = Unbundle By Name(w462) -> ("X"=w461:dbl, "Y"=w460:dbl)
            n350 = local read "WayPoints"() -> (w463:T6[])
            n351 = local read "Units Selector"() -> (w455:T12)
            n352 = in-place {
              in-place-border: w461 -> [w469]
              in-place-border: w460 -> [w468]
              in-place-border: w455 -> [w466]
              n353 = in-place-array #4(w463, w464) -> (w470:T6)
              n354 = in-place {
                in-place-border: w469 -> [w475]
                in-place-border: w468 -> [w474]
                in-place-border: w466 -> [w471]
                n355 = in-place-cluster #5(w470) -> ()  [unwired: 2 out]
                n356 = call "Create_Trajectory_Value_Inches_To_Units.vi"("Units Selector"=w471, "Inches"=w475) -> ("Units"=w472:dbl)  [unwired: 9 in]
                n357 = call "Create_Trajectory_Value_Inches_To_Units.vi"("Units Selector"=w471, "Inches"=w474) -> ("Units"=w473:dbl)  [unwired: 9 in]
                n358 = in-place-cluster #5("X"=w472, "Y"=w473) -> (w467:T6)
              }
              n359 = in-place-array #4(w467) -> (w456:T6[])  [unwired: 1 out]
            }
            n360 = call "Create_Trajectory_All_WP_Units_To_Meters.vi"("Units Selector"=w455, "WayPoints"=w456) -> ("Array"=w454:T6[])  [unwired: 9 in]
            n361 = local write "WayPoints"(w456) -> ()
            n362 = Array Size(array=w454) -> (size(s)=w459:i32)
            n363 = local write "WayPoints_M"(w454) -> ()
            n364 = Greater Or Equal?(x=w459, y=2) -> (x >= y?=w457:bool)
            n365 = case shown="True" w457 {
              frame False {
              }
              frame True {
                n366 = property on="Calculate\nTrajectory" class="Bool (strict)"("Val(Sgnl)"=TRUE ("Value (Signaling)")) -> ()  [unwired: 2 in, 2 out]
              }
            }
          }
          frame False {
          }
        }
      }
      event "Position": Mouse Wheel {
        # "#NOTE Added modifier to allow changing the \nweight if the CTRL key is pressed while moving\nthe mouse wheel."
        # "This gives +/- 1"
        # "Update the waypoint heading....\n\nIf the CTRL key is also pressed\nthen update the weight value \ninstead."
        n367 = event-data() -> ("Delta"=w478:i32, "PlatMods"=w477:T33)  [unwired: 1 in, 8 out]
        n368 = Unbundle By Name(w477) -> ("Ctrl"=w476:bool)
        n369 = local read "Index"() -> (w481:i32)
        n370 = Greater Or Equal To 0?(x=w481) -> (x >= 0?=w480:bool)
        n371 = To Double Precision Float(number=w478) -> (double precision float=w479:dbl)
        n372 = case shown="True" w480 {
          tunnel: w481 -> [w491 _]
          tunnel: w479 -> [w489 _]
          tunnel: w476 -> [w482 _]
          frame True {
            n373 = local read "WayPoints"() -> (w490:T6[])
            n374 = case shown="False" w482 {
              tunnel: w491 -> [w494 w510]
              tunnel: w490 -> [w495 w509]
              tunnel: w489 -> [w493 w508]
              tunnel: [w492 w507] -> w486
              frame True {
                n375 = in-place {
                  in-place-border: w493 -> [w496]
                  n376 = in-place-array #6(w495, w494) -> (w498:T6)
                  n377 = in-place {
                    in-place-border: w496 -> [w501]
                    w505 = 0.01  # Low Limit
                    # "Weight can't be zero."
                    # "Adjust weight"
                    n378 = in-place-cluster #7(w498) -> ("WEIGHT"=w506:dbl)
                    n379 = Multiply(x=0.1, y=w501) -> (x*y=w500:dbl)
                    n380 = Add(x=w506, y=w500) -> (x+y=w503:dbl)
                    n381 = call <vilib>:"MathUtil_Clamp.vi"("High Limit"=inf, "Low Limit"=w505, "Value"=w503) -> ("Result"=w502:dbl)  [unwired: 8 in]
                    n382 = in-place-cluster #7("WEIGHT"=w502) -> (w497:T6)
                  }
                  n383 = in-place-array #6(w497) -> (w492:T6[])  [unwired: 1 out]
                }
              }
              frame False {
                n384 = in-place {
                  in-place-border: w508 -> [w511]
                  n385 = in-place-array #8(w509, w510) -> (w513:T6)
                  n386 = in-place {
                    in-place-border: w511 -> [w518]
                    # "Make it a heading"
                    n387 = in-place-cluster #9(w513) -> ("ANGLE"=w519:dbl)
                    n388 = Add(x=w519, y=w518) -> (x+y=w517:dbl)
                    n389 = call <vilib>:"MathUtil_InputModulus.vi"("Maximum_Input"=180.0, "Minimum_Input"=-180.0, "Input"=w517) -> ("modulus"=w514:dbl)  [unwired: 8 in]
                    n390 = in-place-cluster #9("ANGLE"=w514) -> (w512:T6)
                  }
                  n391 = in-place-array #8(w512) -> (w507:T6[])  [unwired: 1 out]
                }
              }
            }
            n392 = local read "Units Selector"() -> (w483:T12)
            n393 = local write "WayPoints"(w486) -> ()
            n394 = call "Create_Trajectory_All_WP_Units_To_Meters.vi"("Units Selector"=w483, "WayPoints"=w486) -> ("Array"=w484:T6[])  [unwired: 9 in]
            n395 = Array Size(array=w484) -> (size(s)=w485:i32)
            n396 = local write "WayPoints_M"(w484) -> ()
            n397 = Greater Or Equal?(x=w485, y=2) -> (x >= y?=w487:bool)
            n398 = case shown="True" w487 {
              frame False {
              }
              frame True {
                n399 = property on="Calculate\nTrajectory" class="Bool (strict)"("Val(Sgnl)"=TRUE ("Value (Signaling)")) -> ()  [unwired: 2 in, 2 out]
              }
            }
          }
          frame False {
          }
        }
      }
      event "Add New\nWaypoint": Value Change {
        # "If  Index < 0 or index == size-1\n     put at end\nelse"
        # "#TODO   If this is the first then put in the middle of screen.....\n                                    DONE\n                 If not at end then put in the middle of prev and next\n                                    DONE\n                 If new at end  -- if room -- then put X+24, Y, \n                                else put X, Y+/- 24 towards middle.\n                                    NOT DONE - may not really need."
        n400 = event-data() -> ("NewVal"=w521:bool)  [unwired: 1 in, 5 out]
        n401 = case shown="True" w521 {
          frame False {
          }
          frame True {
            # "Add a waypoint after the current one.."
            # "If something selected\nthen add after the\nselected item.  If nothing\nselected add to the end."
            n402 = local read "WayPoints"() -> (w531:T6[])
            n403 = local read "Index"() -> (w530:i32)
            n404 = Greater Or Equal To 0?(x=w530) -> (x >= 0?=w550:bool)
            n405 = Array Size(array=w531) -> (size(s)=w541:i32)
            n406 = local read "Units Selector"() -> (w529:T12)
            n407 = Increment(x=w530) -> (x+1=w548:i32)
            n408 = Decrement(x=w541) -> (x-1=w540:i32)
            n409 = Select(t=w548, s=w550, f=w541) -> (s? t:f=w549:i32)
            n410 = Less?(x=w530, y=w540) -> (x < y?=w538:bool)
            n411 = Greater Or Equal To 0?(x=w530) -> (x >= 0?=w539:bool)
            n412 = Greater Or Equal?(x=w541, y=2) -> (x >= y?=w537:bool)
            n413 = local read "Reverse"() -> (w522:bool)
            n414 = Compound Arithmetic op=AND(w539, w538, w537) -> (w536:bool)
            n415 = case shown="True" w536 {
              tunnel: [315.0 ("X") w574] -> w533
              tunnel: [162.0 ("Y") w573] -> w532
              tunnel: w531 -> [_ w584]
              tunnel: w530 -> [_ w582]
              tunnel: w529 -> [_ w568]
              tunnel: [0.0 ("Y") w570] -> w523
              tunnel: w522 -> [_ w557]
              frame False {
                # "Y inches"
                # "x inches"
                # "Angle  Deg"
                # "Put the cursor\nin the middle of the\nfield."
              }
              frame True {
                w577 = 0.5 ("x")
                # "Ang deg"
                # "Y inch"
                # "X inch"
                # "Put it in the middle of our two\npoints..."
                n416 = Increment(x=w582) -> (x+1=w583:i32)
                n417 = Index Array(array=w584, index #1=w582, index #2=w583) -> (element #1=w581:T6, element #2=w580:T6)
                n418 = Unbundle By Name(w581) -> ("X"=w564:dbl, "Y"=w566:dbl)
                n419 = Unbundle By Name(w580) -> ("X"=w565:dbl, "Y"=w567:dbl)
                n420 = Add(x=w566, y=w567) -> (x+y=w579:dbl)
                n421 = Subtract(x=w567, y=w566) -> (x-y=w563:dbl)
                n422 = Subtract(x=w565, y=w564) -> (x-y=w562:dbl)
                n423 = Add(x=w564, y=w565) -> (x+y=w578:dbl)
                n424 = Inverse Tangent (2 Input)(1:w562, 2:w563) -> (0:w559:dbl)
                n425 = Multiply(x=w577, y=w579) -> (x*y=w576:dbl)
                n426 = Multiply(x=w577, y=w578) -> (x*y=w575:dbl)
                n427 = Add(x=3.141592653589793, y=w559) -> (x+y=w558:dbl)
                n428 = Select(t=w558, s=w557, f=w559) -> (s? t:f=w561:dbl)
                n429 = call "Create_Trajectory_Value_Units_To_Inches.vi"("Units Selector"=w568, "Units"=w575) -> ("Inches"=w574:dbl)  [unwired: 9 in]
                n430 = call "Create_Trajectory_Value_Units_To_Inches.vi"("Units Selector"=w568, "Units"=w576) -> ("Inches"=w573:dbl)  [unwired: 9 in]
                n431 = call <vilib>:"Conv_Radians_Deg.vi"("Radians"=w561) -> ("Degrees"=w569:dbl)  [unwired: 10 in]
                n432 = call <vilib>:"MathUtil_InputModulus.vi"("Maximum_Input"=180.0, "Minimum_Input"=-180.0, "Input"=w569) -> ("modulus"=w570:dbl)  [unwired: 8 in]
              }
            }
            n433 = call "Create_Trajectory_Value_Inches_To_Units.vi"("Units Selector"=w529, "Inches"=w533) -> ("Units"=w544:dbl)  [unwired: 9 in]
            n434 = call "Create_Trajectory_Value_Inches_To_Units.vi"("Units Selector"=w529, "Inches"=w532) -> ("Units"=w543:dbl)  [unwired: 9 in]
            n435 = Bundle By Name(cluster=T19 {"Name"="Cursor", "Color"=915580, "Style"=4, "Point Style"=2, "Name Visible"=FALSE, "Allow Drag"=TRUE, "Cursor Mode"=0, "Plot"=0, "Index"=0, "Position"={"X"=315.0, "Y"=162.0}, "X Scale"=0, "Y Scale"=0, "Watch Plots"=[], "Watch All Plots"=FALSE, "Plot Area"=0, "Label Offset"={"X"=0.0, "Y"=0.0}} ("new element/subarray"), "Position.X"=w533, "Position.Y"=w532) -> (w534:T19)
            n436 = property on="Position" class="XYGraph (strict)"() -> ("CrsrList"=w551:T17)  [unwired: 2 in, 2 out]
            n437 = Bundle By Name(cluster=T6 {"X"=315.0, "Y"=162.0, "ANGLE"=0.0, "WEIGHT"=0.0} ("new element/subarray"), "X"=w544, "Y"=w543, "ANGLE"=w523, "WEIGHT"=0.2) -> (w545:T6)
            n438 = Insert Into Array(array=w531, index=w549, new element=w545) -> (w547:T6[])
            n439 = Insert Into Array(array=w551, index=w549, new element=w534) -> (w552:T17)
            n440 = call "Create_Trajectory_All_WP_Units_To_Meters.vi"("Units Selector"=w529, "WayPoints"=w547) -> ("Array"=w528:T6[])  [unwired: 9 in]
            n441 = local write "Index"(w549) -> ()
            n442 = local write "WayPoints"(w547) -> ()
            n443 = local write "WayPoints_M"(w528) -> ()
            n444 = property on="Position" class="XYGraph (strict)"("CrsrList"=w552) -> ()  [unwired: 2 in, 2 out]
            n445 = Array Size(array=w528) -> (size(s)=w527:i32)
            n446 = Greater Or Equal?(x=w527, y=2) -> (x >= y?=w525:bool)
            n447 = case shown="True" w525 {
              frame False {
              }
              frame True {
                n448 = property on="Calculate\nTrajectory" class="Bool (strict)"("Val(Sgnl)"=TRUE ("Value (Signaling)")) -> ()  [unwired: 2 in, 2 out]
              }
            }
          }
        }
      }
      event "WayPoints": Value Change {
        # "Something was typed into a waypoint value.   I think this means that\na row could have been added or deleted too.....\n\nIn this case just:\n\n -- get all the values\n  -- build the Waypoints_M data\n  -- build all the cursors\n  -- trigger the trajectory be rebuilt (if 2 or more waypoints.)"
        n449 = event-data() -> ()  [unwired: 1 in, 6 out]
        n450 = flat-sequence {
          frame #0 {
            n451 = local read "Units Selector"() -> (w590:T12)
            n452 = call "Create_Trajectory_All_WP_Units_To_Meters.vi"("Units Selector"=w590, "WayPoints"="WayPoints") -> ("Array"=w587:T6[])  [unwired: 9 in]
            n453 = call "Create_Trajectory_All_WP_Meters_To_Units.vi"("Units Selector"=TrajCreateUnitsENUM."Inches", "WayPoints_M"=w587) -> ("outWayPoints_UNITS"=w586:T6[])  [unwired: 9 in]
            n454 = for {
              tunnel: w586 -> [w594] mode=indexing
              tunnel: [w591] -> w589 mode=indexing
              n455 = Unbundle By Name(w594) -> ("X"=w593:dbl, "Y"=w592:dbl)
              n456 = Bundle By Name(cluster=T19 {"Name"="Cursor", "Color"=915580, "Style"=4, "Point Style"=2, "Name Visible"=FALSE, "Allow Drag"=TRUE, "Cursor Mode"=0, "Plot"=0, "Index"=0, "Position"={"X"=315.0, "Y"=162.0}, "X Scale"=0, "Y Scale"=0, "Watch Plots"=[], "Watch All Plots"=FALSE, "Plot Area"=0, "Label Offset"={"X"=0.0, "Y"=0.0}} ("new element/subarray"), "Position.X"=w593, "Position.Y"=w592) -> (w591:T19)
            }
            n457 = local write "WayPoints_M"(w587) -> ()
            n458 = property on="Position" class="XYGraph (strict)"("CrsrList"=w589) -> ()  [unwired: 2 in, 2 out]
          }
          frame #1 {
            n459 = property on="Calculate\nTrajectory" class="Bool (strict)"("Val(Sgnl)"=TRUE ("Value (Signaling)")) -> ()  [unwired: 2 in, 2 out]
          }
        }
      }
      event "Remove Current\nWaypoint": Value Change {
        n460 = event-data() -> ("NewVal"=w597:bool)  [unwired: 1 in, 5 out]
        n461 = case shown="True" w597 {
          frame False {
          }
          frame True {
            # "Only do anyting\nif there is something\nto remove."
            n462 = local read "Index"() -> (w599:i32)
            n463 = Greater Or Equal To 0?(x=w599) -> (x >= 0?=w598:bool)
            n464 = case shown="True" w598 {
              tunnel: w599 -> [_ w600]
              frame False {
              }
              frame True {
                # "Remove cursoe"
                n465 = flat-sequence {
                  tunnel: w600 -> [w610]
                  frame #0 {
                    # "Just in case"
                    # "Remove Waypoint"
                    n466 = local read "WayPoints"() -> (w609:T6[])
                    n467 = property on="Position" class="XYGraph (strict)"() -> ("CrsrList"=w608:T17)  [unwired: 2 in, 2 out]
                    n468 = local read "Units Selector"() -> (w601:T12)
                    n469 = Delete From Array(array=w609, length=1, index=w610) -> (array with subset deleted=w604:T6[])  [unwired: 1 out]
                    n470 = Delete From Array(array=w608, length=1, index=w610) -> (array with subset deleted=w607:T17)  [unwired: 1 out]
                    n471 = local write "WayPoints"(w604) -> ()
                    n472 = call "Create_Trajectory_All_WP_Units_To_Meters.vi"("Units Selector"=w601, "WayPoints"=w604) -> ("Array"=w602:T6[])  [unwired: 9 in]
                    n473 = property on="Position" class="XYGraph (strict)"("CrsrList"=w607) -> ()  [unwired: 2 in, 2 out]
                    n474 = Decrement(x=w610) -> (x-1=w605:i32)
                    n475 = Array Size(array=w602) -> (size(s)=w603:i32)
                    n476 = local write "WayPoints_M"(w602) -> ()
                    n477 = local write "Index"(w605) -> ()
                    n478 = Greater Or Equal?(x=w603, y=2) -> ()  [unwired: 1 out]
                  }
                  frame #1 {
                    # "#NOTE Try and recalc trajectory\neven if there are too few waypoints."
                    n479 = property on="Calculate\nTrajectory" class="Bool (strict)"("Val(Sgnl)"=TRUE ("Value (Signaling)")) -> ()  [unwired: 2 in, 2 out]
                  }
                }
              }
            }
          }
        }
      }
    }
    n480 = case shown="True" "Terminate" {
      frame False {
      }
      frame True {
        # "The end program button was pressed."
        n481 = disable-structure shown="Default" {
          frame condition #0 (active) {
            n482 = Stop(stop? (T)=TRUE) -> ()
          }
          frame condition #1 {
            n483 = Quit LabVIEW(quit? (T)=TRUE) -> ()
          }
        }
      }
    }
  }
